vi "2017RefLoopPulseGen_Summer.vi"() -> ()   [LabVIEW 2017]
uses:
  offset_parameters.ctl
  Utility Sub VIs/pressure_temp_mixture.ctl
  Utility Sub VIs/pulse_generator_multiheater_controls.ctl
  Utility Sub VIs/valve_pid_control.ctl
  Utility Sub VIs/pulse_generator_data.ctl
  Utility Sub VIs/pulse_generator_data_charts.ctl
  Utility Sub VIs/pulse_generator_data_controls.ctl
  Input Channel Lists/test_section_physical_channels.ctl
  Input Channel Lists/float_switch_physical_channels.ctl
  Input Channel Lists/pulse_generator_input_physical_channels.ctl
  Input Channel Lists/pg_control_physical_channels.ctl
  Input Channel Lists/valve_physical_channels.ctl
  Input Channel Lists/window_heater_physical_channels.ctl
  Utility Sub VIs/windows_heater_safety_values.ctl
  Utility Sub VIs/window_heaters_control.ctl
  Utility Sub VIs/visual_loop.ctl
  Utility Sub VIs/diode_charts.ctl
  <vilib>/Utility/error.llb/DialogType.ctl
  Input Channel Lists/label_array_cluster.ctl
  Utility Sub VIs/pulse_generator_controls_multiheater_refnums.ctl
  <vilib>/Utility/sysdir.llb/System Directory Type.ctl
  <vilib>/DAQmx/read.llb/DAQmx Read (Analog 1D Wfm NChan NSamp).vi
  <vilib>/Utility/file.llb/Write Delimited Spreadsheet (string).vi
  <vilib>/DAQmx/configure/timing.llb/DAQmx Timing (Sample Clock).vi
  <vilib>/DAQmx/miscellaneous.llb/DAQmx Fill In Error Info.vi
  Utility Sub VIs/max_flow_correlation.vi
  <vilib>/addons/control/pid/autopid.llb/PID Autotuning.vi
  Stop_Global_Variable.vi
  <resource>/objmgr/daqmx.rc
  <vilib>/dex/Stream Element Allocation Mode.ctl
panel:
  out "notifier out":refnum<notifier>
  out "Float 5":bool
  out "Float 4":bool
  out "Float 3":bool
  out "Float 2":bool
  out "Float 1":bool
  out "Pulse Generator":u8(slide) scale=0.0..100.0 scale format="%.0f%"
  out "Valve Voltage Output":dbl[](array[numeric])
  out "dataQueue":refnum<queue>
  out "autoOffsetPsatQueue":refnum<queue>
  out "start time":timestamp
  out "Seconds Since\nSession Start":dbl
  out "Time Stamp":timestamp format="%<%H:%M:%S%1u>T"
  out "Data Labels":string[][](array[string])
  in  "Tab Control":T1(tab)
  in  "Tabulated/Visualized":enum32{"Tabulated", "Visualized"}(tab)
  in  "Zero Pressure Offsets":bool
  in  "Zero Temp Offsets":bool
  out "Pressure/Temperature/Mixture Properties":T2
  in  "Auto Offset":bool
  in  "Offset Parameters":T3
  out "Auto Offset Progress":u32(slide) scale=0.0..20.0
  out "# of Datasets Processed":i32
  out "Visual Loop Display":T4
  in  "Vapor PID Control":T5={"proportional gain (Kc)"=7.1567, "integral time (Ti, min)"=4.7515, "derivative time (Td, min)"=0.0, "Valve Voltage [V]"=1.0, "Min % Open"=2.0, "Max % Open"=10.0, "Reinitialize?"=FALSE, "Valve On/Off"=FALSE, "Mode"=FALSE, "Full Flow Rate"=-0.0, "Flow Set Point [g/s]"=0.0, "AutoTune"=FALSE, "Flow"={"Flow rate [g/s]"=0.0, "Line Density [g/cm^3]"=0.0}} {"Flow Set Point [g/s]" format="%.2f"; "Full Flow Rate" format="%.2f"; "Max % Open" min=0.0 max=100.0 format="%.2f"; "Min % Open" min=0.0 max=100.0 format="%.2f"; "Valve Voltage [V]" min=1.0 max=5.0 step=0.01 format="%.4f"; "derivative time (Td, min)" format="%.3f"; "integral time (Ti, min)" format="%.3f"; "proportional gain (Kc)" format="%.3f"}
  in  "Liquid PID Control":T5={"proportional gain (Kc)"=7.157, "integral time (Ti, min)"=4.752, "derivative time (Td, min)"=0.0, "Valve Voltage [V]"=1.0, "Min % Open"=2.0, "Max % Open"=3.0, "Reinitialize?"=FALSE, "Valve On/Off"=FALSE, "Mode"=FALSE, "Full Flow Rate"=0.0, "Flow Set Point [g/s]"=0.0, "AutoTune"=FALSE, "Flow"={"Flow rate [g/s]"=0.0, "Line Density [g/cm^3]"=0.0}} {"Flow Set Point [g/s]" format="%.2f"; "Full Flow Rate" format="%.2f"; "Max % Open" min=0.0 max=100.0 format="%.2f"; "Min % Open" min=0.0 max=100.0 format="%.2f"; "Valve Voltage [V]" min=1.0 max=5.0 step=0.01 format="%.4f"; "derivative time (Td, min)" format="%.3f"; "integral time (Ti, min)" format="%.3f"; "proportional gain (Kc)" format="%.3f"}
  out "Vapor Mass Flow Rate":T6(graph)
  out "Liquid Mass Flow Rate":T6(graph)
  in  "Pulse Generator Offsets":T7
  out "Measurements Data":T8={"PG Abs Pressure"=119484.80284900061, "Vapor Temperature"=19.805676371442082, "Liquid Temperature"=19.52526901660894, "TS Temperature W1"=121.24568157832624, "TS Temperature W7"=119.96937909943745, "TS Abs Pressure W1"=121.24568157832624, "TS Abs Pressure W7"=119.96937909943745, "W1-4 dP[Pa]"=19.52526901660894, "W1-7 dP[Pa]"=119.96937909943745, "W1-7 dP[Pa] Fast"=119.96937909943745, "PG Pitot dP [Pa]"=119.96937909943745, "Vapor Line Pitot dP [Pa]"=119.96937909943745, "Vapor Sat Pressure"=121.24568157832624, "Liquid Sat Pressure"=119.96937909943745, "PG Mass Flow Rate"=nan, "Vapor Line Mass Flow"=119.96937909943745}
  out "Pulse Generator Charts":T9={"Vapor Mass Flow Rates"={"max value"=119484.80284900061, "max value"=11360.460004869077}, "Test Section Thermocouples"={"max value"=0.0, "max value"=0.0, "max value"=0.0}, "Pulse Generator Abs Pressure"=[], "Test Section Saturation Pressures"={"max value"=0.0, "max value"=0.0}}
  out "Diode Charts":T10={"Diodes"={0.3021955968100006, 0.3584869363750005}, "Intensity Ratio"=0.8429751997821322, "TS Window 1 Temperatures"={"Average"=20.97750879446322, "T Sat [C]"=14.276809363087821}}
  in  "Commit Settings":bool
  in  "Settings Subpanel":T11(tab)
  in  "Input":T15={"Control Input Physical Channels"={"Vapor Mass Flow Current"="cDAQ1Mod2/ai5", "Vapor Line Density Current"="cDAQ1Mod2/ai6", "Liquid Mass Flow Current"="cDAQ1Mod2/ai3", "Liquid Line Density Current"="cDAQ1Mod2/ai4", "Vapor Tank Pressure"="cDAQ1Mod5/ai1", "Liquid Tank Pressure"="cDAQ1Mod5/ai2", "Separator Pressure"="cDAQ1Mod5/ai0", "Liquid Inlet Pressure"="cDAQ1Mod5/ai4", "Vapor Inlet Pressure"="cDAQ1Mod5/ai3", "Vapor Tank Temperature"="cDAQ1Mod6/ai1", "Vapor Inlet Temperature"="cDAQ1Mod7/ai2", "Liquid Tank Temperature"="cDAQ1Mod6/ai2", "Liquid Inlet Temperature"="cDAQ1Mod7/ai3", "Separator Temperature"="cDAQ1Mod6/ai0", "Lower Dev Section Pressure"="cDAQ1Mod5/ai6", "Test Section Temperature"="cDAQ1Mod6/ai10", "Upper Dev Section Temperature"="cDAQ1Mod6/ai3", "Upper Dev Section Pressure"="cDAQ1Mod5/ai5", "Atmospheric Pressure"="cDAQ1Mod5/ai8", "Mixing Tee dP"="cDAQ1Mod5/ai9", "PG inlet-Mixing Tee Pressure"="cDAQ1Mod5/ai10", "Test Section Pressure"="cDAQ1Mod5/ai7", "PG inlet-Mixing Tee Temperature"="cDAQ1Mod7/ai6"}, "Float Switch Physical Channels"={"Float Line 1"="Input/port0/line0", "Float Line 2"="Input/port0/line1", "Float Line 3"="Input/port0/line2", "Float Line 4"="Input/port0/line3", "Float Line 5"="Input/port0/line4"}, "Measurement Input Physical Channels"={"PG Absolute Pressure"="cDAQ1Mod5/ai11", "Pitot dP"="cDAQ1Mod2/ai7", "PG Temperature 1"="cDAQ1Mod7/ai4", "PG Temperature 2"="cDAQ1Mod7/ai5", "dP Windows 1 to 7"="cDAQ1Mod2/ai2", "dP Windows 1 to 4"="cDAQ1Mod2/ai1", "Camera Voltage"="cDAQ1Mod8/ai0", "dP Windows 1 to 4 F"="cDAQ1Mod2/ai0", "TS Temperature W1"="cDAQ1Mod6/ai4", "TS Temperature W7"="cDAQ1Mod6/ai5", "TS Abs Pressure W1"="cDAQ1Mod5/ai12", "TS Abs Pressure W7"="cDAQ1Mod5/ai13", "Main Diode"="cDAQ1Mod8/ai1", "Temperature Diode"="cDAQ1Mod8/ai2", "TS Exterior Temp"="cDAQ1Mod6/ai6", "DS Exterior Temp"="cDAQ1Mod6/ai7", "Vapor Line Pitot dP"=""}, "Float Switch Line Mode"=TRUE}
  in  "Output":T19={"Pulse Generator Control Physical Channels"={"1000W 1"="Output/port0/line1", "1000W 2"="Output/port0/line2", "1000W 3"="Output/port0/line3", "500W 1"="Output/port0/line4", "250W 1"="Output/port0/line5", "150W 1"="Output/port0/line6", "Counter Line"="cDAQ1Mod1/ctr0", "Direction Line"="cDAQ1Mod1/port0/line1"}, "Proportional Valve Physical Channels"={"Vapor Valve"="cDAQ1Mod3/ao1", "Liquid Valve"="cDAQ1Mod3/ao2", "PG Valve"="cDAQ1Mod3/ao0"}, "Window Heaters Physical Channels"={"On/Off"="cDAQ1Mod4/ao0"}, "Diode Communication"={"URL"="", "Serial"=""}}
  in  "Safety":T21={"Pulse Generator Heater Safety Values"={"Absolute Pulse Generator Pressure Limit"=250000.0, "Seconds Allowed Pulse Generator Excess Pressure"=60.0, "Absolute Pulse Generator Temperature Limit"=35.0}, "Window Heater Safety Values"={"Minimum Test Section Mass Flow "=1.0}}
  in  "Generate MATLAB Parsing Script":bool
  in  "Open Brians VI":bool
  in  "Run Log":T22(array[cluster])
  out "System Running":bool
  out "error out":errorcluster
  out "Loop Time [ms]":u32
  in  "Stop":bool
  in  "Tab Control 2":enum32{"Controls", "Offsets"}(tab)
  in  "Pulse Train, Steam Heater Controls":T23={"Start Pulse"=FALSE, "Stop Pulse"=FALSE, "Pulse Gen\nActive?"=FALSE, "Frequency (Hz)"=3000.0, "Duty Cycle"=0.5, "Idle State"=10214, "Steps"=1000, "Stepper Motor Direction"=FALSE, "Heaters"=FALSE, "Heater ON?"=FALSE, "1000-1"=FALSE, "1000-2"=FALSE, "1000-3"=FALSE, "500-1"=FALSE, "250-1"=FALSE, "150-1"=FALSE, "Valve Voltage [V]"=1.0, "Valve On/Off"=FALSE, "Power [W]"=1.0} {"Power [W]" min=1.0 max=5.0 format="%.2f"; "Valve Voltage [V]" min=1.0 max=5.0 format="%.2f"; "Frequency (Hz)" min=1.0 step=500.0; "Duty Cycle" min=0.1 max=0.99 step=0.1; "Idle State" items=["High"=10192, "Low"=10214]}
  in  "Window Heaters Control":T24
  in  "Data Saving Parameters":T25={"Sampling\nFrequency"=1000.0, "Recording Duration [s]"=10.0, "Data Index"=0, "Data Prefix"="", "Data Folder"=path "C:/Users/rmorse/Desktop/testdata", "Record Data"=FALSE, "Data Recording Progress"=0, "Notes: "=""} {"Data Recording Progress" scale=0.0..10000.0}
  in  "Offsets":T26(array[cluster])
  # "Saturation\nPressure [Pa]"
  # "Saturation\nTemperature [C]"
  # "Pressure [Pa]"
  # "Temperature [C]"
  # "Liquid Tank"
  # "Separator"
  # "Liquid Inlet"
  # "Vapor Tank"
  # "Vapor Inlet"
  # "Test Section"
  # "Upper Dev Section"
  # "Lower Dev Section"
  # "Pulse Gen"
  # "Test Section"
  # "Normal: NC\nInvert: NO\nSwitch 0 is inverted"
  # "NI-9401 Counter & DIO (pin) Chart"
  # "Default Pins used by Counter:\n     SRC: P-Gen Counter Timebase, A-input  \n     GATE: P-Gen Trigger, Z-input\n     AUX: B-input \n     OUT: P_Gen Output\nMore info:  Programs»National Instruments»NI-DAQ»NI-DAQmx Key Concepts»Counters"
  # "0"
  # "1"
  # "2"
  # "3"
  # "7 (25)"
  # "6 (23)"
  # "4 (20)"
  # "5 (22)"
  # "3 (19)"
  # "2 (17)"
  # "0 (14)"
  # "1 (16)"
  # "4 (20)"
  # "5 (22)"
  # "6 (23)"
  # "7 (25)"
  # "0 (14)"
  # "1 (16)"
  # "2 (17)"
  # "3 (19)"
  # "COUNTER"
  # "SRC"
  # "GATE"
  # "AUX"
  # "OUT"
  # "Heater Switches"
  # "PG Valve"
  # "Current Nominal Power"
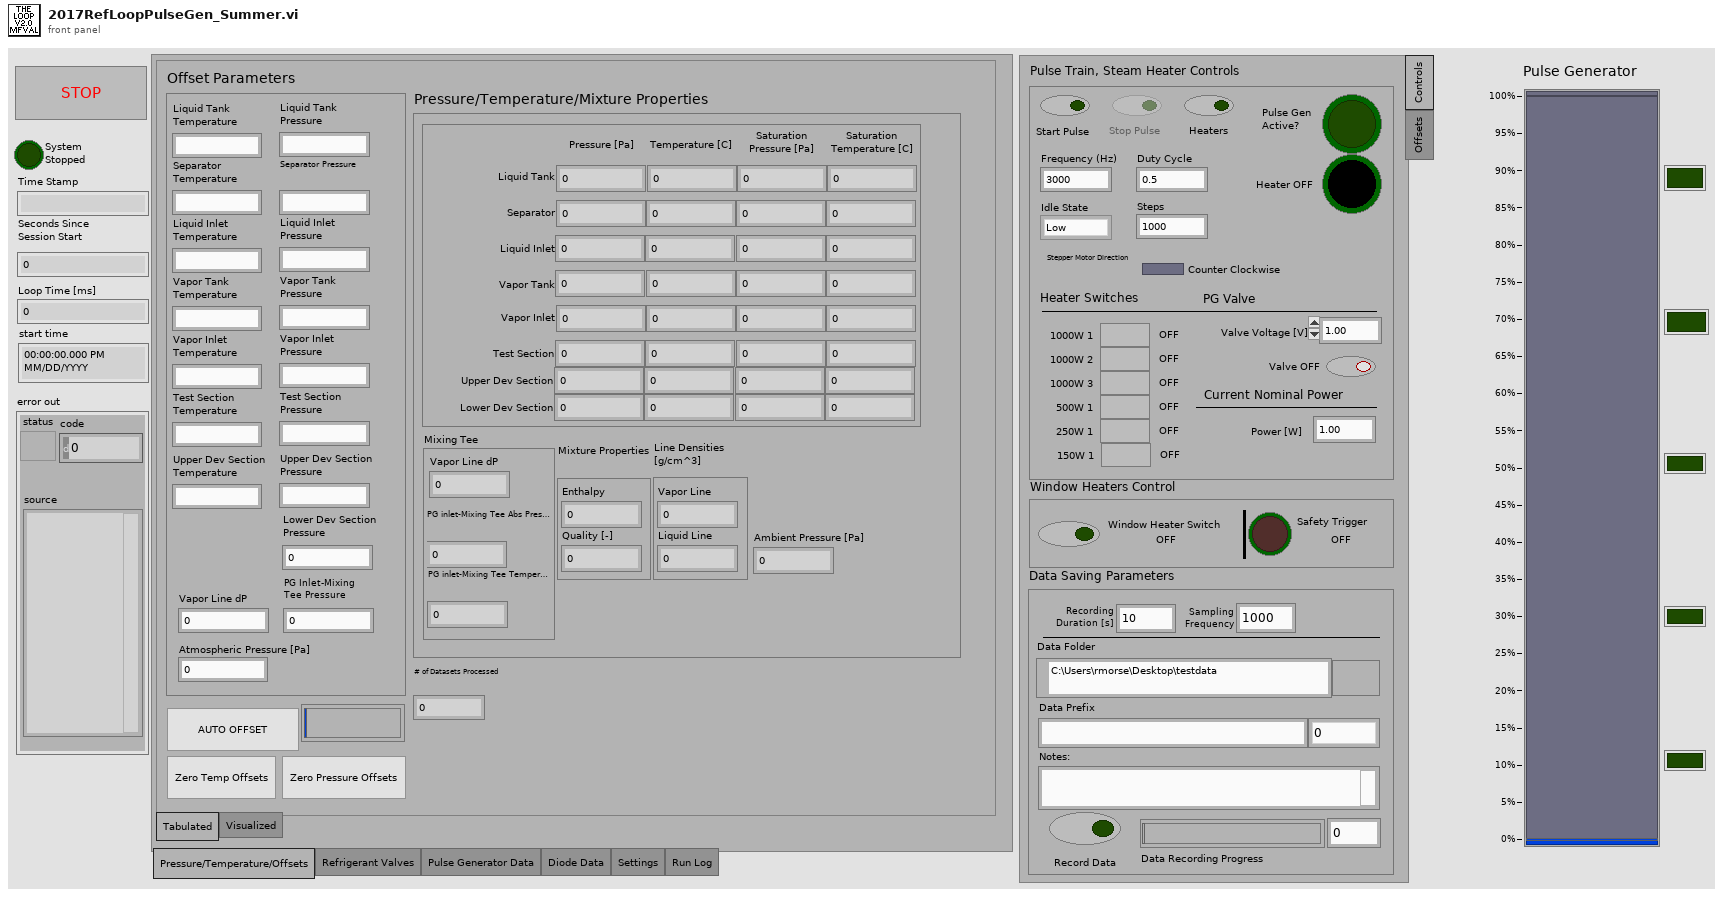
[diagram p1: front panel]
types:
  T1 = enum32{"Pressure/Temperature/Offsets", "Refrigerant Valves", "Pulse Generator Data", "Diode Data", "Settings", "Run Log"}
  T2 = typedef "pressure_temp_mixture.ctl" = cluster{"Line Densities\n[g/cm^3]":cluster{"Vapor Line":dbl, "Liquid Line":dbl}, "Mixture Properties":cluster{"Enthalpy":dbl, "Quality [-]":dbl}, "Component PTs":cluster{"Liquid Tank P":dbl, "Liquid Tank T":dbl, "Liquid Tank Sat P":dbl, "Liquid Tank Sat T":dbl, "Separator P":dbl, "Separator T":dbl, "Separator Sat P":dbl, "Separator Sat T":dbl, "Liquid Inlet P":dbl, "Liquid Inlet T":dbl, "Liquid Inlet Sat P":dbl, "Liquid Inlet Sat T":dbl, "Vapor Tank P":dbl, "Vapor Tank T":dbl, "Vapor Tank Sat P":dbl, "Vapor Tank Sat T":dbl, "Vapor Inlet P":dbl, "Vapor Inlet T":dbl, "Vapor Inlet Sat P":dbl, "Vapor Inlet Sat T":dbl, "Test Section P":dbl, "Test Section T":dbl, "Test Section Sat P":dbl, "Test Section Sat T":dbl, "Upper Dev Section P":dbl, "Upper Dev Section T":dbl, "Upper Dev Section Sat P":dbl, "Upper Dev Section Sat T":dbl, "Lower Dev Section P":dbl, "Lower Dev Section T":dbl, "Lower Dev Section Sat P":dbl, "Lower Dev Section Sat T":dbl}, "Ambient Pressure [Pa]":dbl, "Mixing Tee":cluster{"Vapor Line dP":dbl, "PG inlet-Mixing Tee Abs Pressure":dbl, "PG inlet-Mixing Tee Temperature":dbl}}
  T3 = typedef "offset_parameters.ctl" = cluster{"Liquid Tank\nPressure":dbl, "Liquid Tank\nTemperature":dbl, "Separator Pressure":dbl, "Separator \nTemperature":dbl, "Liquid Inlet\nPressure":dbl, "Liquid Inlet\nTemperature ":dbl, "Vapor Tank\nPressure ":dbl, "Vapor Tank\nTemperature ":dbl, "Vapor Inlet\nPressure":dbl, "Vapor Inlet \nTemperature":dbl, "Test Section\nPressure":dbl, "Test Section\nTemperature":dbl, "Upper Dev Section\nPressure":dbl, "Upper Dev Section\nTemperature":dbl, "Lower Dev Section\nPressure":dbl, "PG Inlet-Mixing Tee Pressure":dbl, "Vapor Line dP":dbl, "Atmospheric Pressure [Pa]":dbl}
  T4 = typedef "visual_loop.ctl" = cluster{"VpTkTemp":dbl, "VpTkPres":dbl, "LiqTkTemp":dbl, "LiqTkPres":dbl, "PGVapTemp":dbl, "PgPres":dbl, "VapInTemp":dbl, "VapInPres":dbl, "SepTemp":dbl, "SepPres":dbl, "TSInTemp":dbl, "TSInPres":dbl, "LiqInTemp":dbl, "LiqInPres":dbl, "DevTemp":dbl, "DevPres":dbl, "TSTemp":dbl, "TSPres":dbl, "Win1-4dP":dbl, "Win1-7dP":dbl, "LiqMass":dbl, "VpMass":dbl, "PGMass":dbl, "PGLiqTemp":dbl}
  T5 = typedef "valve_pid_control.ctl" = cluster{"proportional gain (Kc)":dbl, "integral time (Ti, min)":dbl, "derivative time (Td, min)":dbl, "Valve Voltage [V]":dbl, "Min % Open":dbl, "Max % Open":dbl, "Reinitialize?":bool, "Valve On/Off":bool, "Mode":bool, "Full Flow Rate":dbl, "Flow Set Point [g/s]":dbl, "AutoTune":bool, "Flow":cluster{"Flow rate [g/s]":dbl, "Line Density [g/cm^3]":dbl}}
  T6 = cluster{"Flow Set Point [g/s]":dbl, "Flow rate [g/s]":dbl}
  T7 = typedef "pulse_generator_data_controls.ctl" = cluster{"PG Pitot dP Offset":dbl, "PG Abs Offset":dbl, "W1-7 dP Offset":dbl, "W1-4 dP Offset ":dbl, "TS Abs 1 Offset":dbl, "W1-4 Fast dP Offset":dbl, "TS Abs 2 Offset":dbl, "Vapor Line Pitot dP Offset":dbl}
  T8 = typedef "pulse_generator_data.ctl" = cluster{"PG Abs Pressure":dbl, "Vapor Temperature":dbl, "Liquid Temperature":dbl, "TS Temperature W1":dbl, "TS Temperature W7":dbl, "TS Abs Pressure W1":dbl, "TS Abs Pressure W7":dbl, "W1-4 dP[Pa]":dbl, "W1-7 dP[Pa]":dbl, "W1-7 dP[Pa] Fast":dbl, "PG Pitot dP [Pa]":dbl, "Vapor Line Pitot dP [Pa]":dbl, "Vapor Sat Pressure":dbl, "Liquid Sat Pressure":dbl, "PG Mass Flow Rate":dbl, "Vapor Line Mass Flow":dbl}
  T9 = typedef "pulse_generator_data_charts.ctl" = cluster{"Vapor Mass Flow Rates":cluster{"max value":dbl, "max value":dbl}, "Test Section Thermocouples":cluster{"max value":dbl, "max value":dbl, "max value":dbl}, "Pulse Generator Abs Pressure":dbl[], "Test Section Saturation Pressures":cluster{"max value":dbl, "max value":dbl}}
  T10 = typedef "diode_charts.ctl" = cluster{"Diodes":cluster{dbl, dbl}, "Intensity Ratio":dbl, "TS Window 1 Temperatures":cluster{"Average":dbl, "T Sat [C]":dbl}}
  T11 = enum32{"Input", "Output", "Safety", "Other Functions"}
  T12 = typedef "test_section_physical_channels.ctl" = cluster{"Vapor Mass Flow Current":tag, "Vapor Line Density Current":tag, "Liquid Mass Flow Current":tag, "Liquid Line Density Current":tag, "Vapor Tank Pressure":tag, "Liquid Tank Pressure":tag, "Separator Pressure":tag, "Liquid Inlet Pressure":tag, "Vapor Inlet Pressure":tag, "Vapor Tank Temperature":tag, "Vapor Inlet Temperature":tag, "Liquid Tank Temperature":tag, "Liquid Inlet Temperature":tag, "Separator Temperature":tag, "Lower Dev Section Pressure":tag, "Test Section Temperature":tag, "Upper Dev Section Temperature":tag, "Upper Dev Section Pressure":tag, "Atmospheric Pressure":tag, "Mixing Tee dP":tag, "PG inlet-Mixing Tee Pressure":tag, "Test Section Pressure":tag, "PG inlet-Mixing Tee Temperature":tag}
  T13 = typedef "float_switch_physical_channels.ctl" = cluster{"Float Line 1":tag, "Float Line 2":tag, "Float Line 3":tag, "Float Line 4":tag, "Float Line 5":tag}
  T14 = typedef "pulse_generator_input_physical_channels.ctl" = cluster{"PG Absolute Pressure":tag, "Pitot dP":tag, "PG Temperature 1":tag, "PG Temperature 2":tag, "dP Windows 1 to 7":tag, "dP Windows 1 to 4":tag, "Camera Voltage":tag, "dP Windows 1 to 4 F":tag, "TS Temperature W1":tag, "TS Temperature W7":tag, "TS Abs Pressure W1":tag, "TS Abs Pressure W7":tag, "Main Diode":tag, "Temperature Diode":tag, "TS Exterior Temp":tag, "DS Exterior Temp":tag, "Vapor Line Pitot dP":tag}
  T15 = cluster{"Control Input Physical Channels":T12, "Float Switch Physical Channels":T13, "Measurement Input Physical Channels":T14, "Float Switch Line Mode":bool}
  T16 = typedef "pg_control_physical_channels.ctl" = cluster{"1000W 1":tag, "1000W 2":tag, "1000W 3":tag, "500W 1":tag, "250W 1":tag, "150W 1":tag, "Counter Line":tag, "Direction Line":tag}
  T17 = typedef "valve_physical_channels.ctl" = cluster{"Vapor Valve":tag, "Liquid Valve":tag, "PG Valve":tag}
  T18 = typedef "window_heater_physical_channels.ctl" = cluster{"On/Off":tag}
  T19 = cluster{"Pulse Generator Control Physical Channels":T16, "Proportional Valve Physical Channels":T17, "Window Heaters Physical Channels":T18, "Diode Communication":cluster{"URL":string, "Serial":refnum<visa-resource-name>}}
  T20 = typedef "windows_heater_safety_values.ctl" = cluster{"Minimum Test Section Mass Flow ":dbl}
  T21 = cluster{"Pulse Generator Heater Safety Values":cluster{"Absolute Pulse Generator Pressure Limit":dbl, "Seconds Allowed Pulse Generator Excess Pressure":dbl, "Absolute Pulse Generator Temperature Limit":dbl}, "Window Heater Safety Values":T20}
  T22 = cluster{"File Number":string, "Entry Content":string}[]
  T23 = typedef "pulse_generator_multiheater_controls.ctl" = cluster{"Start Pulse":bool, "Stop Pulse":bool, "Pulse Gen\nActive?":bool, "Frequency (Hz)":dbl, "Duty Cycle":dbl, "Idle State":i32, "Steps":i32, "Stepper Motor Direction":bool, "Heaters":bool, "Heater ON?":bool, "1000-1":bool, "1000-2":bool, "1000-3":bool, "500-1":bool, "250-1":bool, "150-1":bool, "Valve Voltage [V]":dbl, "Valve On/Off":bool, "Power [W]":dbl}
  T24 = typedef "window_heaters_control.ctl" = cluster{"Window Heater Switch":bool, "Safety Trigger":bool}
  T25 = cluster{"Sampling\nFrequency":dbl, "Recording Duration [s]":dbl, "Data Index":i32, "Data Prefix":string, "Data Folder":path, "Record Data":bool, "Data Recording Progress":u32, "Notes: ":string}
  T26 = cluster{"Channel":string, "Offset":dbl, "Output Unit":enum16{"psi", "Pa", "inH2O", "inHg", "C", "K", "g/s", "g/cm3", "Volt", "Amp", ""}}[]
  T27 = enum32{"Pressure/Temperature/Offsets", "Refrigerant Valves", "Pulse Generator Data", "Diode Data", "Settings"}
  T28 = enum8{"Enabled", "Disabled", "Disabled and Grayed Out"}
  T29 = cluster{"max value":dbl, "max value":dbl, "max value":dbl}[]
  T30 = enum32{"Pressure/Temperature/Offsets", "Refrigerant Valves", "Pulse Generator Data", "Settings"}
  T31 = cluster{"Channel Name":string, "Label":string, "Offset":dbl, "Raw":dbl[], "Processed":dbl[], "Converted":dbl[], "Average":dbl}
  T32 = typedef "label_array_cluster.ctl" = cluster{"Label Array":string[]}
  T33 = enum32{"Invalid", "Standard", "Closed", "Hidden", "Minimized", "Maximized"}
  T34 = cluster{"Entry Content":string, "File Number":string}
  T35 = typedef "DialogType.ctl" = u16
  T36 = cluster{"Flow Set Point [g/s]":dbl, "Flow rate [g/s]":dbl}[]
  T37 = typedef "analog_data_channel_pkg.ctl" = cluster{"Analog Input Channel":T38, "Analog Data":T39}
  T38 = typedef "input_channel.ctl" = cluster{"Channel Name":string, "Physical Channel":tag, "Sensor Type":enum16{"Absolute Pressure", "Gauge Pressure", "Differential Pressure", "Temperature", "Mass Flow Rate", "Density", "Other"}, "Signal Type":enum16{"Voltage", "Current", "Temperature"}, "Terminal Configuration":i32, "Minimum Value":dbl, "Maximum Value":dbl, "TC Type":i32, "Sensor Min":dbl, "Sensor Max":dbl, "Sensor Offset":dbl, "Sensor Unit":enum16{"psi", "Pa", "inH2O", "inHg", "C", "K", "g/s", "g/cm3", "Volt", "Amp", ""}, "Output Unit":enum16{"psi", "Pa", "inH2O", "inHg", "C", "K", "g/s", "g/cm3", "Volt", "Amp", ""}, "Unit Conversion":dbl, "Active":bool, "Input Type":enum16{"DAQ", "Add-On"}}
  T39 = typedef "analog_data.ctl" = cluster{"Label":string, "Offset":dbl, "Raw":dbl[], "Converted":dbl[], "Average":dbl, "Formula To Output":string, "Formula From Output":string}
  T40 = enum16{"psi", "Pa", "inH2O", "inHg", "C", "K", "g/s", "g/cm3", "Volt", "Amp", ""}
  T41 = cluster{"Label":string, "Offset":dbl, "Output Unit":enum16{"psi", "Pa", "inH2O", "inHg", "C", "K", "g/s", "g/cm3", "Volt", "Amp", ""}}
  T42 = typedef "index_array_cluster.ctl" = cluster{"Index Array":i32[]}
  T43 = typedef "Stream Element Allocation Mode.ctl" = u32
  T44 = typedef "pulse_generator_controls_multiheater_refnums.ctl" = cluster{"Start Pulse":refnum<vi>, "Stop Pulse":refnum<vi>, "Heaters":refnum<vi>, "Counter":refnum<vi>, "Frequency (Hz)":refnum<vi>, "Duty Cycle":refnum<vi>, "Idle State":refnum<vi>, "Pulse Generator Active":refnum<vi>, "Stepper Motor Direction":refnum<vi>, "Steps":refnum<vi>, "Direction Line":refnum<vi>, "1000-1 Line":refnum<vi>, "1000-2 Line":refnum<vi>, "1000-3 Line":refnum<vi>, "500-1 Line":refnum<vi>, "250-1 Line":refnum<vi>, "1000-1":refnum<vi>, "1000-2":refnum<vi>, "1000-3":refnum<vi>, "500-1":refnum<vi>, "250-1":refnum<vi>, "150-1":refnum<vi>, "Heater ON?":refnum<vi>, "150-1 Line":refnum<vi>, "Power":refnum<vi>}
  T45 = cluster{"Liquid Tank P":dbl, "Liquid Tank T":dbl, "Liquid Tank Sat P":dbl, "Liquid Tank Sat T":dbl, "Separator P":dbl, "Separator T":dbl, "Separator Sat P":dbl, "Separator Sat T":dbl, "Liquid Inlet P":dbl, "Liquid Inlet T":dbl, "Liquid Inlet Sat P":dbl, "Liquid Inlet Sat T":dbl, "Vapor Tank P":dbl, "Vapor Tank T":dbl, "Vapor Tank Sat P":dbl, "Vapor Tank Sat T":dbl, "Vapor Inlet P":dbl, "Vapor Inlet T":dbl, "Vapor Inlet Sat P":dbl, "Vapor Inlet Sat T":dbl, "Test Section P":dbl, "Test Section T":dbl, "Test Section Sat P":dbl, "Test Section Sat T":dbl, "Upper Dev Section P":dbl, "Upper Dev Section T":dbl, "Upper Dev Section Sat P":dbl, "Upper Dev Section Sat T":dbl, "Lower Dev Section P":dbl, "Lower Dev Section T":dbl, "Lower Dev Section Sat P":dbl, "Lower Dev Section Sat T":dbl}
  T46 = cluster{"Channel":string, "Offset":dbl, "Output Unit":enum16{"psi", "Pa", "inH2O", "inHg", "C", "K", "g/s", "g/cm3", "Volt", "Amp", ""}}
  T47 = typedef "System Directory Type.ctl" = i32
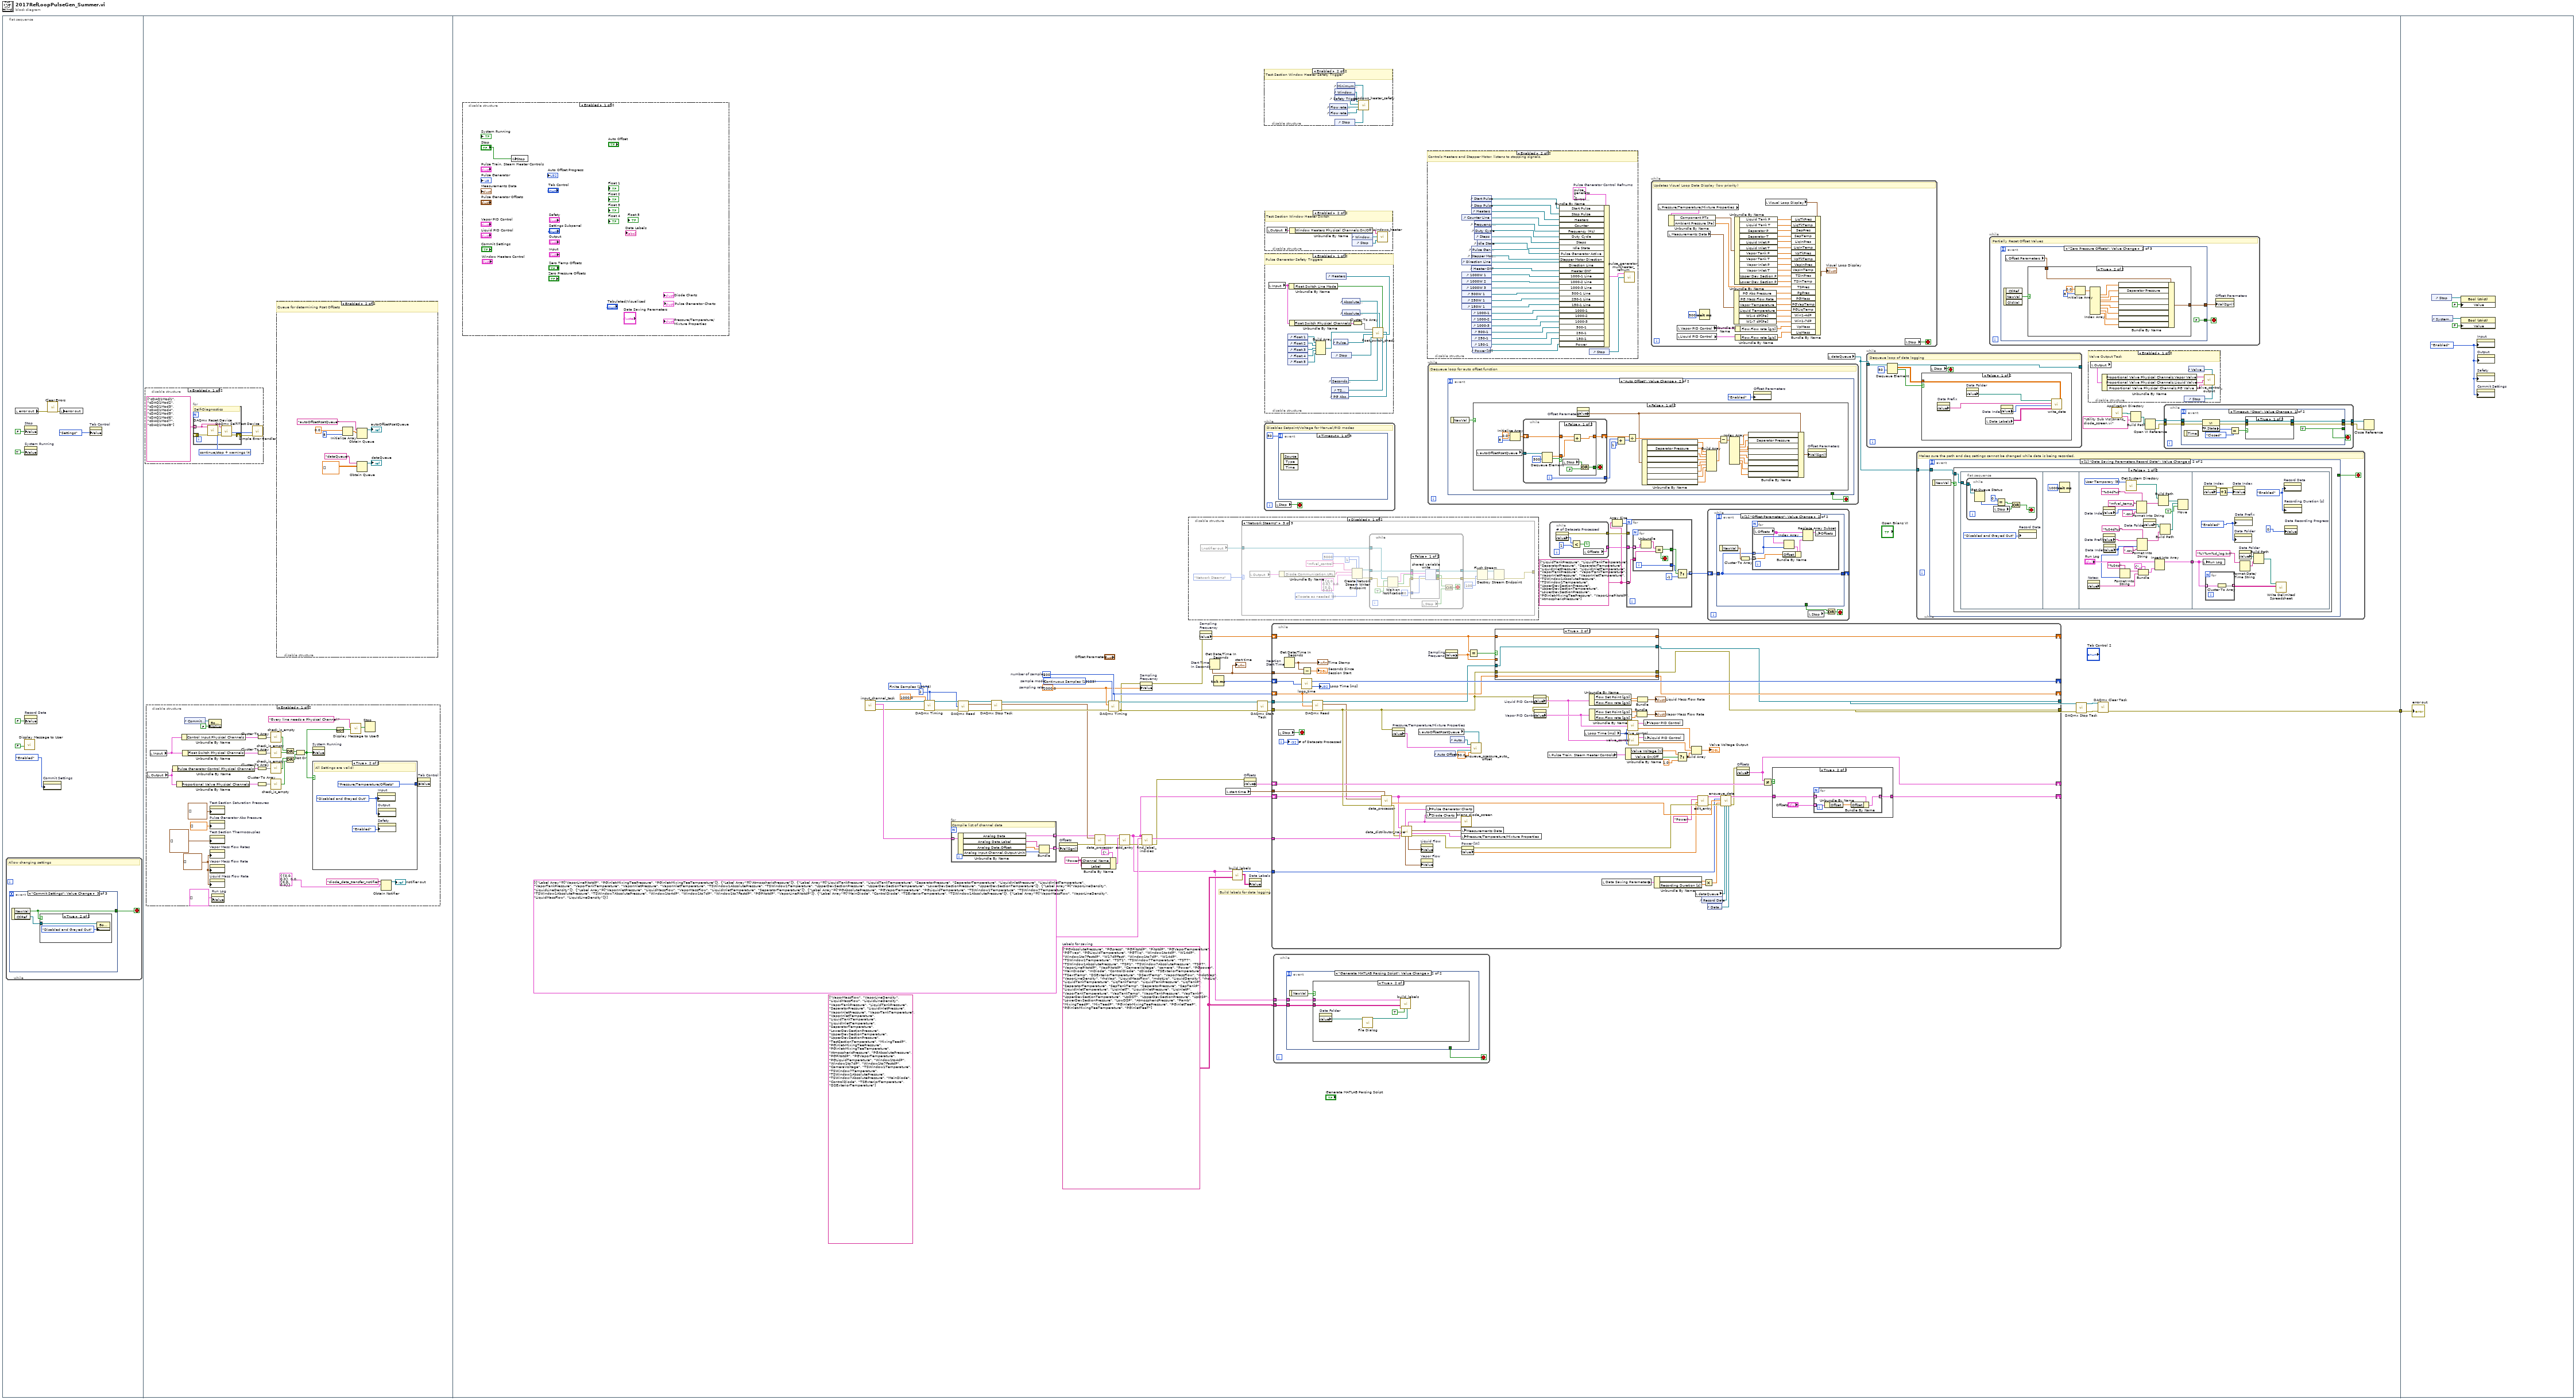
[diagram p0: block diagram]
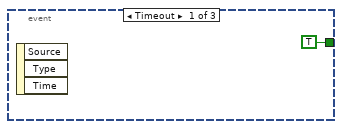
[diagram p2: hidden frame]
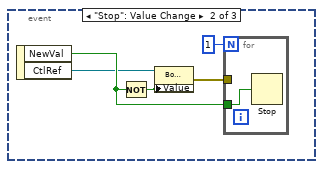
[diagram p3: hidden frame]
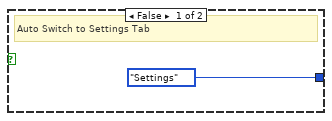
[diagram p6: hidden frame]
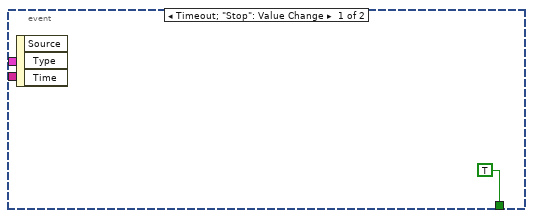
[diagram p9: hidden frame]
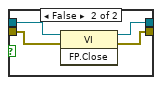
[diagram p11: hidden frame]
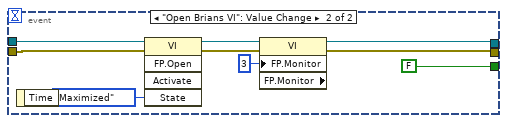
[diagram p12: hidden frame]
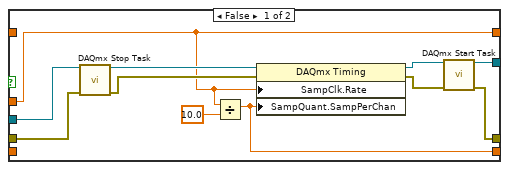
[diagram p14: hidden frame]
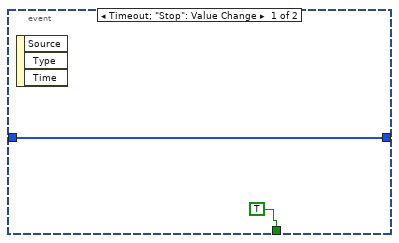
[diagram p15: hidden frame]
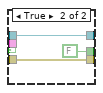
[diagram p18: hidden frame]
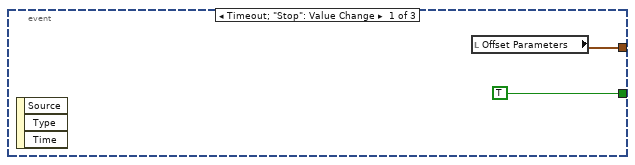
[diagram p20: hidden frame]
diagram:
  n1 = flat-sequence {
    tunnel: [w130] -> w1
    tunnel: w1 -> [w628]
    frame #0 {
      n2 = while {
        stop <- w10 stop-if-true
        # "Allow changing settings"
        n3 = event shown="[2] \"Commit Settings\": Value Change" {
          selector: _ -> [_ _ _]
          dyn-events: _ -> [_ _ _]
          timeout: _ -> [_ _ _]
          tunnel: [TRUE ("NewVal") _ w18] -> w10
          event Timeout {
            n4 = event-data() -> ()  [unwired: 1 in, 3 out]
          }
          event "Stop": Value Change {
            n5 = event-data() -> ("NewVal"=w16:bool, "CtlRef"=w15:refnum<vi>)  [unwired: 1 in]
            n6 = Not(x=w16) -> (.not. x?=w14:bool)
            n7 = property class="Bool (strict)"(reference=w15, "Value"=w14) -> (error out=w13:errorcluster)  [unwired: 1 in, 1 out]
            n8 = for {
              N: 1 -> [_]
              tunnel: w16 -> [w17]
              tunnel: w13 -> [_]
              n9 = Stop(stop? (T)=w17) -> ()
            }
          }
          event "Commit Settings": Value Change {
            n10 = event-data() -> ("NewVal"=w18:bool, "CtlRef"=w19:refnum<vi>)  [unwired: 1 in]
            n11 = case shown="True" w18 {
              tunnel: w19 -> [_ w21]
              frame False {
              }
              frame True {
                n12 = property class="Bool (strict)"(reference=w21, "DisabledEnum"=T28."Disabled and Grayed Out" ("Disabled")) -> ()  [unwired: 1 in, 2 out]
              }
            }
          }
        }
      }
      n13 = local read "error out"() -> (w9:errorcluster)
      n14 = call "Display Message to User"("Enable"=FALSE) -> ()  [unwired: 9 in, 2 out]
      n15 = property on="Stop" class="Bool (strict)"("Value"=FALSE) -> ()  [unwired: 2 in, 2 out]
      n16 = property on="System Running" class="Bool (strict)"("Value"=TRUE) -> ()  [unwired: 2 in, 2 out]
      n17 = property on="Record Data" class="Bool (strict)"("Value"=FALSE) -> ()  [unwired: 2 in, 2 out]
      n18 = property on="Commit Settings" class="Bool (strict)"("DisabledEnum"=T28."Enabled" ("Disabled")) -> ()  [unwired: 2 in, 2 out]
      n19 = call <vilib>:"Clear Errors.vi"("error in (no error)"=w9) -> ("error out"=w7:errorcluster)  [unwired: 5 in, 1 out]
      n20 = local write "error out"(w7) -> ()
      n21 = property on="Tab Control" class="TabCtl (strict)"("Value"=T27."Settings" ("Tab Control")) -> ()  [unwired: 2 in, 2 out]
    }
    frame #1 {
      n22 = disable-structure shown="Enabled" {
        frame Enabled {
          w65 = T35 4 items=["no dialog", "OK message", "continue or stop message", "OK message + warnings", "continue/stop + warnings"] ("type of dialog (OK msg:1)")
          n23 = for {
            tunnel: string[] ["cDAQ1Mod1", "cDAQ1Mod2", "cDAQ1Mod3", "cDAQ1Mod4", "cDAQ1Mod5", "cDAQ1Mod6", "cDAQ1Mod7", "cDAQ1Mod8"] -> [w69] mode=indexing
            shift-right: [w71] -> w66
            shift-left: _ -> [w68]
            # "Self-Diagnostics"
            n24 = call <vilib>:"DAQmx Reset Device.vi"("device in"=w69, "error in"=w68) -> ("error out"=w70:errorcluster)  [unwired: 13 in]
            n25 = call <vilib>:"DAQmx Self-Test Device.vi"("device in"=w69, "error in"=w70) -> ("error out"=w71:errorcluster)  [unwired: 13 in]
          }
          n26 = call <vilib>:"Simple Error Handler.vi"("type of dialog (OK msg:1)"=w65, "error in (no error)"=w66) -> ()  [unwired: 3 in, 5 out]
        }
        frame Disabled {
        }
      }
      n27 = disable-structure shown="Enabled" {
        frame Enabled {
          w31 = T36 [] ("History Data")
          n28 = local read "Output"() -> (w38:T19)
          n29 = local read "Input"() -> (w44:T15)
          n30 = Unbundle By Name(w38) -> ("Pulse Generator Control Physical Channels"=w45:T16)
          n31 = Unbundle By Name(w38) -> ("Proportional Valve Physical Channels"=w43:T17)
          n32 = Unbundle By Name(w44) -> ("Control Input Physical Channels"=w47:T12)
          n33 = Unbundle By Name(w44) -> ("Float Switch Physical Channels"=w46:T13)
          n34 = control-ref of="Commit Settings"() -> (w41:refnum<vi>)
          n35 = property class="Bool (strict)"(reference=w41, "Value"=FALSE ("Commit Settings")) -> ()  [unwired: 1 in, 2 out]
          n36 = property on="Test Section Saturation Pressures" class="WFChart (strict)"("History Data"=cluster{"max value":dbl, "max value":dbl}[] []) -> ()  [unwired: 2 in, 2 out]
          n37 = property on="Pulse Generator Abs Pressure" class="WFChart (strict)"("History Data"=dbl[] []) -> ()  [unwired: 2 in, 2 out]
          n38 = property on="Test Section Thermocouples" class="WFChart (strict)"("History Data"=T29 []) -> ()  [unwired: 2 in, 2 out]
          n39 = property on="Vapor Mass Flow Rates" class="WFChart (strict)"("History Data"=w31) -> ()  [unwired: 2 in, 2 out]
          n40 = property on="Vapor Mass Flow Rate" class="WFChart (strict)"("History Data"=w31) -> ()  [unwired: 2 in, 2 out]
          n41 = property on="Liquid Mass Flow Rate" class="WFChart (strict)"("History Data"=w31) -> ()  [unwired: 2 in, 2 out]
          n42 = property on="Run Log" class="Arr (strict)"("Value"=T22 [] ("Run Log")) -> ()  [unwired: 2 in, 2 out]
          n43 = Cluster To Array(cluster=w47) -> (array=w60:tag[])
          n44 = Cluster To Array(cluster=w46) -> (array=w59:tag[])
          n45 = Cluster To Array(cluster=w45) -> (array=w56:tag[])
          n46 = Cluster To Array(cluster=w43) -> (array=w54:tag[])
          n47 = call "check_is_empty.vi"("Channels"=w60) -> ("Has Empty?"=w58:bool)
          n48 = call "check_is_empty.vi"("Channels"=w59) -> ("Has Empty?"=w57:bool)
          n49 = call "check_is_empty.vi"("Channels"=w56) -> ("Has Empty?"=w53:bool)
          n50 = call "check_is_empty.vi"("Channels"=w54) -> ("Has Empty?"=w52:bool)
          n51 = Or(x=w58, y=w57) -> (x .or. y?=w55:bool)
          n52 = Or(x=w53, y=w52) -> (x .or. y?=w51:bool)
          n53 = Not Or(1:w51, 2:w55) -> (0:w39:bool)
          n54 = property on="System Running" class="Bool (strict)"("Value"=w39) -> ()  [unwired: 2 in, 2 out]
          n55 = case shown="True" w39 {
            tunnel: [T30."Settings" ("Tab Control") T27."Pressure/Temperature/Offsets" ("Tab Control")] -> w42
            frame False {
              # "Auto Switch to Settings Tab"
            }
            frame True {
              w63 = T28."Disabled and Grayed Out" ("Disabled")
              # "All Settings are valid!"
              n56 = property on="Input" class="Clust (strict)"("DisabledEnum"=w63) -> ()  [unwired: 2 in, 2 out]
              n57 = property on="Output" class="Clust (strict)"("DisabledEnum"=w63) -> ()  [unwired: 2 in, 2 out]
              n58 = property on="Safety" class="Clust (strict)"("DisabledEnum"=T28."Enabled" ("Disabled")) -> ()  [unwired: 2 in, 2 out]
            }
          }
          n59 = Not(x=w39) -> (.not. x?=w50:bool)
          n60 = call "Display Message to User5"("Enable"=w50, "Message"="Every line needs a Physical Channel!") -> ("OK"=w48:bool)  [unwired: 8 in, 1 out]
          n61 = Stop(stop? (T)=w48) -> ()
          n62 = Obtain Notifier(name (unnamed)="diode_data_transfer_notifier", notification data type=T10 {"Diodes"={0.0, 0.0}, "Intensity Ratio"=0.0, "TS Window 1 Temperatures"={"Average"=0.0, "T Sat [C]"=0.0}} ("Diode Charts")) -> (notifier out=→"notifier out":refnum<notifier>)  [unwired: 2 in, 2 out]
          n63 = property on="Tab Control" class="TabCtl (strict)"("Value"=w42) -> ()  [unwired: 2 in, 2 out]
        }
        frame Disabled {
        }
      }
      n64 = disable-structure shown="Enabled" {
        frame Disabled {
        }
        frame Enabled {
          # "Queue for determining Psat Offsets"
          n65 = Initialize Array(0.0 ("element"), 8 ("dimension size")) -> (w29:dbl[])
          n66 = Obtain Queue(name (unnamed)="autoOffsetPsatQueue", element data type=w29) -> (queue out=→"autoOffsetPsatQueue":refnum<queue>)  [unwired: 3 in, 2 out]
          n67 = Obtain Queue(name (unnamed)="dataQueue", element data type=dbl[][] [] ("appended array")) -> (queue out=→"dataQueue":refnum<queue>)  [unwired: 3 in, 2 out]
        }
      }
    }
    frame #2 {
      w84 = "Power" ("Channel Name")
      w102 = 10178 items=["Finite Samples"=10178, "Continuous Samples"=10123, "Hardware Timed Single Point"=12522] ("sample mode")
      w98 = 2 ("samples per channel")
      w110 = string[] ["LiquidTankPressure", "LiquidTankTemperature", "SeparatorPressure", "SeparatorTemperature", "LiquidInletPressure", "LiquidInletTemperature", "VaporTankPressure", "VaporTankTemperature", "VaporInletPressure", "VaporInletTemperature", "TSWindow1AbsolutePressure", "TSWindow1Temperature", "UpperDevSectionPressure", "UpperDevSectionTemperature", "LowerDevSectionPressure", "PGinlet-MixingTeePressure", "VaporLinePitotdP", "AtmosphericPressure"] ("Array")
      w73 = string[][] [["PGAbsolutePressure", "PGpress"], ["PGPitotdP", "PitotdP"], ["PGVaporTemperature", "PGTvap"], ["PGLiquidTemperature", "PGTliq"], ["Window1to4dP", "W14dP"], ["Window1to7FastdP", "W17dPFast"], ["Window1to7dP", "W14dP"], ["TSWindow1Temperature", "TST1"], ["TSWindow7Temperature", "TST7"], ["TSWindow1AbsolutePressure", "TSP1"], ["TSWindow7AbsolutePressure", "TSP7"], ["VaporLinePitotdP", "VapPitotdP"], ["CameraVoltage", "camera"], ["Power", "PGpower"], ["MainDiode", "mDiode"], ["ControlDiode", "cDiode"], ["TSExteriorTemperature", "TSextTemp"], ["DSExteriorTemperature", "DSextTemp"], ["VaporMassFlow", "mdotVap"], ["VaporLineDensity", "rhoVap"], ["LiquidMassFlow", "mdotLiq"], ["LiquidDensity", "rhoLiq"], ["LiquidTankTemperature", "LiqTankTemp"], ["LiquidTankPressure", "LiqTankP"], ["SeparatorTemperature", "SepTankTemp"], ["SeparatorPressure", "SepTankP"], ["LiquidInletTemperature", "LiqInletT"], ["LiquidInletPressure", "LiqInletP"], ["VaporTankTemperature", "VapTankTemp"], ["VaporTankPressure", "VapTankP"], ["UpperDevSectionTemperature", "UpDST"], ["UpperDevSectionPressure", "UpDSP"], ["LowerDevSectionPressure", "LowDSP"], ["AtmosphericPressure", "Pamb"], ["MixingTeedP", "MixTeedP"], ["PGinlet-MixingTeePressure", "PGinletTeeP"], ["PGinlet-MixingTeeTemperature", "PGinletTeeT"]]  # Labels for saving
      (unwired) string[] ["VaporMassFlow", "VaporLineDensity", "LiquidMassFlow", "LiquidLineDensity", "VaporTankPressure", "LiquidTankPressure", "SeparatorPressure", "LiquidInletPressure", "VaporInletPressure", "VaporTankTemperature", "VaporInletTemperature", "LiquidTankTemperature", "LiquidInletTemperature", "SeparatorTemperature", "LowerDevSectionPressure", "UpperDevSectionTemperature", "UpperDevSectionPressure", "TestSectionTemperature", "MixingTeedP", "PGinlet-MixingTeePressure", "PGinlet-MixingTeeTemperature", "AtmosphericPressure", "PGAbsolutePressure", "PGPitotdP", "PGVaporTemperature", "PGLiquidTemperature", "Window1to4dP", "Window1to7dP", "Window1to7FastdP", "CameraVoltage", "TSWindow1Temperature", "TSWindow7Temperature", "TSWindow1AbsolutePressure", "TSWindow7AbsolutePressure", "MainDiode", "ControlDiode", "TSExteriorTemperature", "DSExteriorTemperature"] ("Array")
      w125 = 10123 items=["Finite Samples"=10178, "Continuous Samples"=10123, "Hardware Timed Single Point"=12522]  # sample mode
      w123 = 2000.0  # sampling rate
      w124 = 200  # number of samples
      # "Build labels for data logging"
      n68 = disable-structure shown="Enabled" {
        frame Enabled {
          n69 = global write "Stop_Global_Variable.vi" "Stop"("Stop") -> ()
        }
        frame Disabled {
        }
      }
      n70 = call "input_channel_task.vi"() -> ("error out"=w103:errorcluster, "Active Analog Channel-Data Packages"=w119:T37[], "task out"=w104:refnum<k21>)  [unwired: 9 in]
      n71 = call-poly <vilib>:"DAQmx Timing.vi"("task/channels in"=w104, "sample mode"=w102, "samples per channel"=w98, "rate"=1000.0, "error in"=w103) -> ("task out"=w100:refnum<k21>, "error out"=w99:errorcluster)  [unwired: 9 in]
      n72 = for {
        tunnel: w119 -> [w311] mode=indexing
        tunnel: [w310] -> w77 mode=indexing
        tunnel: [w308] -> w116 mode=indexing
        # "Compile list of channel data"
        n73 = Unbundle By Name(w311) -> ("Analog Data"=w310:T39, "Analog Data.Label"=w306:string, "Analog Data.Offset"=w309:dbl, "Analog Input Channel.Output Unit"=w307:T40)
        n74 = Bundle("Label"=w306, "Offset"=w309, "Output Unit"=w307) -> (w308:T41)  [unwired: 1 in]
      }
      n75 = call-poly <vilib>:"DAQmx Read.vi"("task/channels in"=w100, "number of samples per channel"=w98, "error in"=w99) -> ("task out"=w97:refnum<k21>, "data"=w78:waveform(dbl)[], "error out"=w96:errorcluster)  [unwired: 10 in]
      n76 = call <vilib>:"DAQmx Stop Task.vi"("task/channels in"=w97, "error in"=w96) -> ("task out"=w94:refnum<k21>, "error out"=w95:errorcluster)  [unwired: 12 in]
      n77 = property on="Offsets" class="Arr (strict)"("Val(Sgnl)"=w116) -> (error out=w80:errorcluster)  [unwired: 2 in, 1 out]
      n78 = Bundle By Name(cluster=T31 {"Channel Name"="", "Label"="", "Offset"=0.0, "Raw"=[], "Processed"=[], "Converted"=[], "Average"=0.0} ("Add-on Data"), "Channel Name"=w84, "Label"=w84) -> (w85:T31)
      n79 = call "data_processor.vi"("Active Analog Data Packages In"=w77, "data"=w78, "error in"=w80) -> ("Analog Data Array"=w83:T39[], "error out"=w82:errorcluster)  [unwired: 10 in, 1 out]
      n80 = call-poly <vilib>:"DAQmx Timing.vi"("task/channels in"=w94, "sample mode"=w125, "samples per channel"=w124, "rate"=w123, "error in"=w95) -> ("task out"=w114:refnum<k21>, "error out"=w113:errorcluster)  [unwired: 9 in]
      n81 = call "add_entry.vi"("Active Analog Data In"=w83, "Add-on Data"=w85, "error in"=w82) -> ("Active Analog Data Out"=w72:T39[], "error out"=w81:errorcluster)  [unwired: 11 in]
      n82 = property on="Sampling\nFrequency" class="DigNum (strict)"(error in=w113, "Value"=w123) -> (error out=w121:errorcluster)  [unwired: 1 in, 1 out]
      n83 = call "find_label_indicies.vi"("error in"=w81, "Array"=T32[] [{"Label Array"=["VaporLinePitotdP", "PGinlet-MixingTeePressure", "PGinlet-MixingTeeTemperature"]}, {"Label Array"=["AtmosphericPressure"]}, {"Label Array"=["LiquidTankPressure", "LiquidTankTemperature", "SeparatorPressure", "SeparatorTemperature", "LiquidInletPressure", "LiquidInletTemperature", "VaporTankPressure", "VaporTankTemperature", "VaporInletPressure", "VaporInletTemperature", "TSWindow1AbsolutePressure", "TSWindow1Temperature", "UpperDevSectionPressure", "UpperDevSectionTemperature", "LowerDevSectionPressure", "UpperDevSectionTemperature"]}, {"Label Array"=["VaporLineDensity", "LiquidLineDensity"]}, {"Label Array"=["VaporInletPressure", "LiquidMassFlow", "VaporMassFlow", "LiquidInletTemperature", "SeparatorTemperature"]}, {"Label Array"=["PGAbsolutePressure", "PGVaporTemperature", "PGLiquidTemperature", "TSWindow1Temperature", "TSWindow7Temperature", "TSWindow1AbsolutePressure", "TSWindow7AbsolutePressure", "Window1to4dP", "Window1to7dP", "Window1to7FastdP", "PGPitotdP", "VaporLinePitotdP"]}, {"Label Array"=["MainDiode", "ControlDiode", "TSExteriorTemperature", "TSWindow1AbsolutePressure"]}, {"Label Array"=["VaporMassFlow", "VaporLineDensity", "LiquidMassFlow", "LiquidLineDensity"]}], "haystack"=w72) -> ("error out"=w79:errorcluster, "Indicies"=w118:T42[])  [unwired: 6 in, 1 out]
      n84 = disable-structure shown="Disabled" {
        frame Disabled {
          n85 = local read "notifier out"() -> (w312:refnum<notifier>)
          n86 = case shown="\"Network Steams\"" enum16{"Network Steams", "Datasocket", "Serial"}."Network Steams" {
            tunnel: w312 -> [_ _ w315]
            tunnel: [_ _ w314] -> _
            frame Default {
            }
            frame "Datasocket" {
            }
            frame "Network Steams" {
              w324 = T43 0 items=["allocate as needed", "pre-allocate"] ("element allocation mode")
              n87 = local read "Output"() -> (w328:T19)
              n88 = Unbundle By Name(w328) -> ("Diode Communication.URL"=w327:string)
              n89 = Create Network Stream Writer Endpoint(5:5000 ("timeout in ms (-1)"), 6:w324, 7:1 ("writer buffer size"), 9:T10 {"Diodes"={0.0, 0.0}, "Intensity Ratio"=0.0, "TS Window 1 Temperatures"={"Average"=0.0, "T Sat [C]"=0.0}} ("Diode Charts"), 10:w327, 11:"mfval_control" ("writer name")) -> (0:w316:errorcluster, 3:w317:refnum<k21>)  [unwired: 1 in]
              n90 = while {
                tunnel: w315 -> [w336]
                tunnel: w317 -> [w339]
                tunnel: [w341] -> w319
                tunnel: w316 -> [w338]
                tunnel: [w340] -> w318
                stop <- w332 stop-if-true
                n91 = Wait on Notification(notifier=w336, ignore previous (F)=TRUE, error in (no error)=w338) -> (notification=w334:T10, timed out?=w333:bool, error out=w337:errorcluster)  [unwired: 1 in, 1 out]
                n92 = case shown="False" w333 {
                  tunnel: 80 ("timeout ms (-1)") -> [w349 _]
                  tunnel: [w348 w352] -> w341
                  tunnel: [w347 w351] -> w340
                  tunnel: w339 -> [w346 w352]
                  tunnel: [w345 FALSE] -> w331
                  tunnel: w337 -> [w344 w351]
                  tunnel: w334 -> [w343 _]
                  frame False {
                    n93 = shared-variable-write(w346, w344, w343, w349) -> (w348:refnum<k21>, w347:errorcluster, w345:bool)
                  }
                  frame True {
                  }
                }
                n94 = local read "Stop"() -> (w330:bool)
                n95 = Or(x=w331, y=w330) -> (x .or. y?=w332:bool)
              }
              n96 = Flush Stream(8:w318, 9:100 ("timeout in ms (-1)"), 11:w319) -> (0:w321:errorcluster, 3:w320:refnum<k21>)  [unwired: 1 in, 1 out]
              n97 = Destroy Stream Endpoint(8:w321, 11:w320) -> (0:w314:errorcluster)
            }
          }
        }
        frame Enabled {
        }
      }
      n98 = property on="Sampling\nFrequency" class="DigNum (strict)"(error in=w121) -> ("Value"=w122:dbl)  [unwired: 1 in, 2 out]
      n99 = Get Date/Time In Seconds "Start Time\nIn Seconds"() -> (seconds since 1Jan1904=w126:timestamp)
      "start time" <- w126
      n100 = Tick Count (ms)() -> (millisecond timer value=w131:u32)
      n101 = local read "start time"() -> (w120:timestamp)
      n102 = call "build_labels.vi"("Labels for saving"=w73, "Analog Data Array In"=w72) -> ("Labels"=w88:string[][], "Label Indicies"=w87:i32[])  [unwired: 8 in]
      n103 = property on="Offsets" class="Arr (strict)"(error in=w79) -> ("Value"=w115:T26)  [unwired: 1 in, 2 out]
      n104 = property on="Data Labels" class="Arr (strict)"("Value"=w88) -> ()  [unwired: 2 in, 2 out]
      n105 = call <vilib>:"DAQmx Start Task.vi"("task/channels in"=w114, "error in"=w113) -> ("task out"=w106:refnum<k21>, "error out"=w105:errorcluster)  [unwired: 12 in]
      n106 = while {
        stop <- w485 stop-if-true
        # "Disables Setpoint/Voltage for Manual/PID modes"
        n107 = local read "Stop"() -> (w485:bool)
        n108 = event shown="[0] Timeout" {
          selector: _ -> [_ _ _]
          dyn-events: _ -> [_ _ _]
          timeout: 50 -> [_ _ _]
          event Timeout {
            n109 = event-data() -> ()  [unwired: 1 in, 3 out]
          }
          event Value Change {
            n110 = event-data() -> ("NewVal"=w487:bool)  [unwired: 1 in]
            n111 = case shown="False" w487 {
              frame False {
                n112 = control-ref of="Valve Voltage [V]"() -> (w491:refnum<vi>)
                n113 = property class="DigNum (strict)"(reference=w491, "DisabledEnum"=T28."Enabled" ("Disabled")) -> ()  [unwired: 1 in, 2 out]
                n114 = control-ref of="Flow Set Point [g/s]"() -> (w489:refnum<vi>)
                n115 = property class="DigNum (strict)"(reference=w489, "DisabledEnum"=T28."Disabled and Grayed Out" ("Disabled")) -> ()  [unwired: 1 in, 2 out]
              }
              frame True {
                n116 = property on="Valve Voltage [V]" class="DigNum (strict)"("DisabledEnum"=T28."Disabled and Grayed Out" ("Disabled")) -> ()  [unwired: 2 in, 2 out]
                n117 = property on="Flow Set Point [g/s]" class="DigNum (strict)"("DisabledEnum"=T28."Enabled" ("Disabled")) -> ()  [unwired: 2 in, 2 out]
              }
            }
          }
          event Value Change {
            n118 = event-data() -> ("NewVal"=w494:bool)  [unwired: 1 in]
            n119 = case shown="False" w494 {
              frame False {
                n120 = control-ref of="Valve Voltage [V]"() -> (w498:refnum<vi>)
                n121 = property class="DigNum (strict)"(reference=w498, "DisabledEnum"=T28."Enabled" ("Disabled")) -> ()  [unwired: 1 in, 2 out]
                n122 = control-ref of="Flow Set Point [g/s]"() -> (w496:refnum<vi>)
                n123 = property class="DigNum (strict)"(reference=w496, "DisabledEnum"=T28."Disabled and Grayed Out" ("Disabled")) -> ()  [unwired: 1 in, 2 out]
              }
              frame True {
                n124 = control-ref of="Valve Voltage [V]"() -> (w502:refnum<vi>)
                n125 = control-ref of="Flow Set Point [g/s]"() -> (w501:refnum<vi>)
                n126 = property class="DigNum (strict)"(reference=w501, "DisabledEnum"=T28."Enabled" ("Disabled")) -> ()  [unwired: 1 in, 2 out]
                n127 = property class="DigNum (strict)"(reference=w502, "DisabledEnum"=T28."Disabled and Grayed Out" ("Disabled")) -> ()  [unwired: 1 in, 2 out]
              }
            }
          }
        }
      }
      n128 = disable-structure shown="Enabled" {
        frame Disabled {
        }
        frame Enabled {
          # "Test Section Window Heater Safety Trigger"
          n129 = control-ref of="Flow rate [g/s]"() -> (w433:refnum<vi>)
          n130 = control-ref of="Flow rate [g/s]"() -> (w432:refnum<vi>)
          n131 = control-ref of="Window Heater Switch"() -> (w436:refnum<vi>)
          n132 = control-ref of="Safety Trigger"() -> (w437:refnum<vi>)
          n133 = control-ref of="Stop"() -> (w434:refnum<vi>)
          n134 = control-ref of="Minimum Test Section Mass Flow"() -> (w435:refnum<vi>)
          n135 = call "windows_heater_safety.vi"("Stop!"=w434, "Minimum Flow Rate Refnum"=w435, "Liquid Flow Rate Refnum"=w432, "Vapor Flow Rate Refnum"=w433, "Safety Trigger Refnum"=w437, "Switch Refnum"=w436) -> ()  [unwired: 1 in]
        }
      }
      n136 = disable-structure shown="Enabled" {
        frame Enabled {
          # "Pulse Generator Safety Triggers"
          n137 = local read "Input"() -> (w468:T15)
          n138 = control-ref of="Float 1"() -> (w484:refnum<vi>)
          n139 = control-ref of="Float 2"() -> (w482:refnum<vi>)
          n140 = control-ref of="Float 3"() -> (w481:refnum<vi>)
          n141 = control-ref of="Float 4"() -> (w483:refnum<vi>)
          n142 = control-ref of="Float 5"() -> (w471:refnum<vi>)
          n143 = Unbundle By Name(w468) -> ("Float Switch Line Mode"=w467:bool)
          n144 = Unbundle By Name(w468) -> ("Float Switch Physical Channels"=w470:T13)
          n145 = Build Array(w484, w482, w481, w483, w471) -> (w480:refnum<vi>[])
          n146 = control-ref of="Heaters"() -> (w477:refnum<vi>)
          n147 = control-ref of="Stop"() -> (w478:refnum<vi>)
          n148 = control-ref of="Seconds Allowed Pulse Generator Excess Pressure"() -> (w474:refnum<vi>)
          n149 = control-ref of="TS Temperature W1"() -> (w472:refnum<vi>)
          n150 = control-ref of="PG Abs Pressure"() -> (w476:refnum<vi>)
          n151 = control-ref of="Pulse Generator"() -> (w479:refnum<vi>)
          n152 = control-ref of="Absolute Pulse Generator Pressure Limit"() -> (w475:refnum<vi>)
          n153 = control-ref of="Absolute Pulse Generator Temperature Limit"() -> (w473:refnum<vi>)
          n154 = Cluster To Array(cluster=w470) -> (array=w469:tag[])
          n155 = call "float_switch_check.vi"("Temperature Refnum"=w472, "Heater Refnum"=w477, "Abs Pressure Refnum"=w476, "InvertLines"=w467, "Abs Temperature Limit Refnum"=w473, "Timeout Refnum"=w474, "Abs Pressure Limit Refnum"=w475, "STOP! Refnum"=w478, "Pulse Generator Slide Refnum"=w479, "Float Indicator Refnum"=w480, "lines array"=w469) -> ()
        }
        frame Disabled {
        }
      }
      n156 = disable-structure shown="Enabled" {
        frame Disabled {
        }
        frame Enabled {
          # "Test Section Window Heater Switch"
          n157 = local read "Output"() -> (w431:T19)
          n158 = Unbundle By Name(w431) -> ("Window Heaters Physical Channels.On/Off"=w428:tag)
          n159 = control-ref of="Window Heater Switch"() -> (w430:refnum<vi>)
          n160 = control-ref of="Stop"() -> (w429:refnum<vi>)
          n161 = call "windows_heater.vi"("Stop! Refnum"=w429, "Switch Refnum"=w430, "Window Heater Switch"=w428) -> ()  [unwired: 1 in]
        }
      }
      n162 = while {
        tunnel: w106 -> [w250]
        tunnel: w105 -> [w249]
        shift-right: [w242] -> _
        shift-left: w131 -> [w243]
        tunnel: w126 -> [w245]
        tunnel: [w232] -> w108
        tunnel: [w233] -> w107
        shift-right: [w238] -> _
        shift-left: w122 -> [w239]
        shift-right: [w234] -> _
        shift-left: w124 -> [w235]
        tunnel: w120 -> [w231]
        shift-right: [w228] -> _
        shift-left: w72 -> [w175]
        tunnel: w118 -> [w206]
        shift-right: [w177] -> _
        shift-left: w115 -> [w229]
        tunnel: w87 -> [w184]
        i -> [w247]
        stop <- w248 stop-if-true
        n163 = local read "Stop"() -> (w248:bool)
        n164 = Get Date/Time In Seconds "Iteration\nStart Time"() -> (seconds since 1Jan1904=w246:timestamp)
        "Time Stamp" <- w246
        n165 = call "loop_time.vi"("previous timer value"=w243) -> ("millisecond timer value"=w242:u32, "Loop Time [ms]"=→"Loop Time [ms]":u32)
        n166 = Subtract(x=w246, y=w245) -> (x-y=→"Seconds Since\nSession Start":dbl)
        n167 = call-poly <vilib>:"DAQmx Read.vi"("task/channels in"=w250, "number of samples per channel"=w235, "error in"=w249) -> ("task out"=w236:refnum<k21>, "data"=w174:waveform(dbl)[], "error out"=w230:errorcluster)  [unwired: 10 in]
        n168 = call "data_processor.vi"("Active Analog Data Packages In"=w175, "start time"=w231, "data"=w174, "error in"=w230) -> ("Analog Data Array"=w179:T39[], "timestamp"=w201:dbl[], "error out"=w200:errorcluster)  [unwired: 9 in]
        n169 = property on="Pressure/Temperature/Mixture Properties" class="Clust (strict)"(error in=w230) -> ("Value"=w207:T2)  [unwired: 1 in, 2 out]
        n170 = call "data_distributor_naive.vi"("error in"=w200, "Indicies"=w206, "Analog Data Array In"=w179) -> ("error out"=w197:errorcluster, "Pressure/Temperature/Mixture Properties"=w183:T2, "Measurements Data"=w182:T8, "Liquid Flow"=w195:cluster{"Average":dbl, "Average":dbl}, "Diode Charts"=w198:T10, "Vapor Flow"=w196:cluster{"Average":dbl, "Average":dbl}, "Pulse Generator Charts"=w199:T9)  [unwired: 2 in]
        n171 = local read "autoOffsetPsatQueue"() -> (w211:refnum<queue>)
        n172 = property on="Liquid Flow" class="Clust (strict)"("Value"=w195) -> ()  [unwired: 2 in, 2 out]
        n173 = property on="Vapor Flow" class="Clust (strict)"("Value"=w196) -> ()  [unwired: 2 in, 2 out]
        n174 = local write "Pulse Generator Charts"(w199) -> ()
        n175 = local write "Diode Charts"(w198) -> ()
        n176 = control-ref of="Auto Offset"() -> (w210:refnum<vi>)
        n177 = property on="Sampling\nFrequency" class="DigNum (strict)"() -> ("Value"=w237:dbl)  [unwired: 2 in, 2 out]
        n178 = control-ref of="Auto Offset Progress"() -> (w208:refnum<vi>)
        n179 = call "brians_diode_screen.vi"("Diode Charts In"=w198) -> ()
        n180 = local write "Measurements Data"(w182) -> ()
        n181 = local write "Pressure/Temperature/Mixture Properties"(w183) -> ()
        n182 = property on="Power [W]" class="DigNum (strict)"(error in=w197) -> (error out=w193:errorcluster, "Value"=w180:dbl)  [unwired: 1 in, 1 out]
        n183 = Equal?(x=w239, y=w237) -> (x = y?=w240:bool)
        n184 = call "enqueue_pressure_auto_offset.vi"("autoOffsetPsatQueue"=w211, "# to average"=30.0, "Auto Offset"=w210, "Pressure/Temperature/Mixture Properties"=w207, "Auto Offset ProgressBar"=w208) -> ()
        n185 = case shown="True" w240 {
          tunnel: w239 -> [_ w273]
          tunnel: [w265 w273] -> w238
          tunnel: w237 -> [w265 _]
          tunnel: w236 -> [w269 w272]
          tunnel: w230 -> [w268 w271]
          tunnel: [w261 w272] -> w233
          tunnel: [w260 w271] -> w232
          tunnel: w235 -> [_ w270]
          tunnel: [w259 w270] -> w234
          frame False {
            n186 = call <vilib>:"DAQmx Stop Task.vi"("task/channels in"=w269, "error in"=w268) -> ("task out"=w267:refnum<k21>, "error out"=w266:errorcluster)  [unwired: 12 in]
            n187 = Divide(x=w265, y=10.0) -> (x/y=w259:dbl)
            n188 = property class="DAQmx Timing"(reference=w267, error in=w266, "SampClk.Rate"=w265, "SampQuant.SampPerChan"=w259) -> (reference out=w263:refnum<k21>, error out=w262:errorcluster)
            n189 = call <vilib>:"DAQmx Start Task.vi"("task/channels in"=w263, "error in"=w262) -> ("task out"=w261:refnum<k21>, "error out"=w260:errorcluster)  [unwired: 12 in]
          }
          frame True {
          }
        }
        n190 = property on="Liquid PID Control" class="Clust (strict)"(error in=w230) -> (error out=w212:errorcluster, "Value"=w220:T5)  [unwired: 1 in, 1 out]
        n191 = property on="Vapor PID Control" class="Clust (strict)"(error in=w212) -> ("Value"=w221:T5)  [unwired: 1 in, 2 out]
        n192 = local read "Pulse Train, Steam Heater Controls"() -> (w214:T23)
        n193 = local read "Loop Time [ms]"() -> (w213:u32)
        n194 = Unbundle By Name(w220) -> ("Flow Set Point [g/s]"=w226:dbl, "Flow.Flow rate [g/s]"=w225:dbl)
        n195 = Unbundle By Name(w221) -> ("Flow Set Point [g/s]"=w224:dbl, "Flow.Flow rate [g/s]"=w223:dbl)
        n196 = local read "Data Saving Parameters"() -> (w190:T25)
        n197 = Unbundle By Name(w214) -> ("Valve Voltage [V]"=w205:dbl, "Valve On/Off"=w204:bool)
        n198 = call "valve_control.vi"("Loop Time [ms]"=w213, "PID Control"=w221) -> ("Valve Voltage [V]"=w218:dbl, "PID Control Output"=w216:T5)  [unwired: 1 in]
        n199 = call "valve_control.vi"("Loop Time [ms]"=w213, "PID Control"=w220) -> ("Valve Voltage [V]"=w217:dbl, "PID Control Output"=w215:T5)  [unwired: 1 in]
        n200 = Bundle("Flow Set Point [g/s]"=w224, "Flow rate [g/s]"=w223) -> (→"Vapor Mass Flow Rate":T6)  [unwired: 1 in]
        n201 = Bundle("Flow Set Point [g/s]"=w226, "Flow rate [g/s]"=w225) -> (→"Liquid Mass Flow Rate":T6)  [unwired: 1 in]
        n202 = local write "Vapor PID Control"(w216) -> ()
        n203 = local write "Liquid PID Control"(w215) -> ()
        n204 = Unbundle By Name(w190) -> ("Sampling\nFrequency"=w192:dbl, "Recording Duration [s]"=w191:dbl)
        n205 = Select(t=w205, s=w204, f=1.0) -> (s? t:f=w202:dbl)
        n206 = Build Array(w218, w217, w202) -> (→"Valve Voltage Output":dbl[])
        n207 = local read "dataQueue"() -> (w189:refnum<queue>)
        n208 = call "edit_entry.vi"("error in"=w193, "Average"=w180, "Label"="Power", "Active Analog Data In"=w179) -> ("error out"=w194:errorcluster, "Active Analog Data Out"=w178:T39[])  [unwired: 5 in]
        n209 = control-ref of="Record Data"() -> (w188:refnum<vi>)
        n210 = Multiply(x=w192, y=w191) -> (x*y=w186:dbl)
        n211 = control-ref of="Data Recording Progress"() -> (w187:refnum<vi>)
        n212 = call "enqueue_data.vi"("Active Analog Data In"=w178, "Label indicies In"=w184, "timestamp"=w201, "# of Samples"=w186, "error in"=w194, "data Queue"=w189, "Record dP Data"=w188, "dP Recording Progress"=w187) -> ("error out"=w176:errorcluster)  [unwired: 7 in]
        n213 = property on="Offsets" class="Arr (strict)"(error in=w176) -> ("Value"=w177:T26)  [unwired: 1 in, 2 out]
        n214 = Not Equal?(x=w177, y=w229) -> (x != y?=w185:bool)
        n215 = case shown="True" w185 {
          tunnel: w178 -> [w251 w252]
          tunnel: [w251 w253] -> w228
          frame False {
          }
          frame True {
            n216 = for {
              tunnel: "Offsets" -> [w257] mode=indexing
              tunnel: [w258] -> w253 mode=indexing
              tunnel: w252 -> [w255] mode=indexing
              n217 = Unbundle By Name(w257) -> ("Offset"=w256:dbl)
              n218 = Bundle By Name(cluster=w255, "Offset"=w256) -> (w258:T39)
            }
          }
        }
        "# of Datasets Processed" <- w247
      }
      n219 = while {
        tunnel: w73 -> [w133]
        tunnel: w72 -> [w132]
        stop <- w134 stop-if-true
        n220 = event shown="[1] \"Generate MATLAB Parsing Script\": Value Change" {
          selector: _ -> [_ _]
          dyn-events: _ -> [_ _]
          timeout: _ -> [_ _]
          tunnel: [TRUE _] -> w134
          tunnel: w133 -> [_ w137]
          tunnel: w132 -> [_ w136]
          event Timeout; "Stop": Value Change {
            n221 = event-data() -> ()  [unwired: 1 in, 3 out]
          }
          event "Generate MATLAB Parsing Script": Value Change {
            n222 = event-data() -> ("NewVal"=w138:bool)  [unwired: 1 in]
            n223 = case shown="True" w138 {
              tunnel: w137 -> [_ w142]
              tunnel: w136 -> [_ w141]
              frame False {
              }
              frame True {
                n224 = property on="Data Folder" class="Path"() -> ("Value"=w140:path)  [unwired: 2 in, 2 out]
                n225 = call "File Dialog"("start path"=w140) -> ("selected path"=w139:path)  [unwired: 11 in, 3 out]
                n226 = call "build_labels.vi"("MATLAB File Directory"=w139, "Save MATLAB Parser?"=TRUE, "Labels for saving"=w142, "Analog Data Array In"=w141) -> ()  [unwired: 6 in, 2 out]
              }
            }
          }
        }
      }
      n227 = disable-structure shown="Enabled" {
        frame Disabled {
        }
        frame Enabled {
          w449 = T44 {"Start Pulse"=refnum, "Stop Pulse"=refnum, "Heaters"=refnum, "Counter"=refnum, "Frequency (Hz)"=refnum, "Duty Cycle"=refnum, "Idle State"=refnum, "Pulse Generator Active"=refnum, "Stepper Motor Direction"=refnum, "Steps"=refnum, "Direction Line"=refnum, "1000-1 Line"=refnum, "1000-2 Line"=refnum, "1000-3 Line"=refnum, "500-1 Line"=refnum, "250-1 Line"=refnum, "1000-1"=refnum, "1000-2"=refnum, "1000-3"=refnum, "500-1"=refnum, "250-1"=refnum, "150-1"=refnum, "Heater ON?"=refnum, "150-1 Line"=refnum, "Power"=refnum}  # Pulse Generator Control Refnums
          # "Controls Heaters and Stepper Motor, listens to stopping signals."
          n228 = control-ref of="Counter Line"() -> (w440:refnum<vi>)
          n229 = control-ref of="Direction Line"() -> (w441:refnum<vi>)
          n230 = control-ref of="1000W 1"() -> (w459:refnum<vi>)
          n231 = control-ref of="1000W 2"() -> (w465:refnum<vi>)
          n232 = control-ref of="1000W 3"() -> (w460:refnum<vi>)
          n233 = control-ref of="500W 1"() -> (w461:refnum<vi>)
          n234 = control-ref of="250W 1"() -> (w462:refnum<vi>)
          n235 = control-ref of="150W 1"() -> (w448:refnum<vi>)
          n236 = control-ref of="Start Pulse"() -> (w455:refnum<vi>)
          n237 = control-ref of="Stop Pulse"() -> (w454:refnum<vi>)
          n238 = control-ref of="Heaters"() -> (w450:refnum<vi>)
          n239 = control-ref of="Pulse Gen\nActive?"() -> (w452:refnum<vi>)
          n240 = control-ref of="Stepper Motor Direction"() -> (w451:refnum<vi>)
          n241 = control-ref of="Heater ON?"() -> (w458:refnum<vi>)
          n242 = control-ref of="1000-1"() -> (w464:refnum<vi>)
          n243 = control-ref of="1000-2"() -> (w463:refnum<vi>)
          n244 = control-ref of="1000-3"() -> (w466:refnum<vi>)
          n245 = control-ref of="500-1"() -> (w447:refnum<vi>)
          n246 = control-ref of="250-1"() -> (w446:refnum<vi>)
          n247 = control-ref of="150-1"() -> (w445:refnum<vi>)
          n248 = control-ref of="Power [W]"() -> (w439:refnum<vi>)
          n249 = control-ref of="Frequency (Hz)"() -> (w453:refnum<vi>)
          n250 = control-ref of="Duty Cycle"() -> (w444:refnum<vi>)
          n251 = control-ref of="Steps"() -> (w443:refnum<vi>)
          n252 = control-ref of="Idle State"() -> (w442:refnum<vi>)
          n253 = Bundle By Name(cluster=w449, "Start Pulse"=w455, "Stop Pulse"=w454, "Heaters"=w450, "Counter"=w440, "Frequency (Hz)"=w453, "Duty Cycle"=w444, "Steps"=w443, "Idle State"=w442, "Pulse Generator Active"=w452, "Stepper Motor Direction"=w451, "Direction Line"=w441, "Heater ON?"=w458, "1000-1 Line"=w459, "1000-2 Line"=w465, "1000-3 Line"=w460, "500-1 Line"=w461, "250-1 Line"=w462, "150-1 Line"=w448, "1000-1"=w464, "1000-2"=w463, "1000-3"=w466, "500-1"=w447, "250-1"=w446, "150-1"=w445, "Power"=w439) -> (w456:T44)
          n254 = control-ref of="Stop"() -> (w457:refnum<vi>)
          n255 = call "pulse_generator_multiheater_refnum.vi"("Stop! Refnum"=w457, "Pulse Generator Control Multiheater Refnums"=w456) -> ()  [unwired: 2 in]
        }
      }
      n256 = while {
        stop <- w503 stop-if-true
        # "Dequeue loop for auto offset function"
        n257 = event shown="[1] \"Auto Offset\": Value Change" {
          selector: _ -> [_ _]
          dyn-events: _ -> [_ _]
          timeout: _ -> [_ _]
          tunnel: [TRUE _] -> w503
          event Timeout; "Stop": Value Change {
            n258 = event-data() -> ()  [unwired: 1 in, 3 out]
          }
          event "Auto Offset": Value Change {
            n259 = event-data() -> ("NewVal"=w506:bool)  [unwired: 1 in]
            n260 = case shown="False" w506 {
              frame False {
                n261 = local read "autoOffsetPsatQueue"() -> (w535:refnum<queue>)
                n262 = Initialize Array(0.0 ("element"), 8 ("dimension size")) -> (w514:dbl[])
                n263 = while {
                  tunnel: w535 -> [w543]
                  shift-right: [w538] -> w534
                  shift-left: w514 -> [w539]
                  tunnel: [w537] -> w532
                  i -> [w537]
                  stop <- w541 stop-if-true
                  n264 = Dequeue Element(queue=w543, timeout in ms (-1)=500) -> (element=w540:dbl[], timed out?=w542:bool)  [unwired: 1 in, 2 out]
                  n265 = case shown="False" w542 {
                    selector: w542 -> [_ w551]
                    tunnel: [w544 w551] -> w541
                    tunnel: w540 -> [w548 _]
                    tunnel: [w547 w550] -> w538
                    tunnel: w539 -> [w549 w550]
                    frame False {
                      n266 = local read "Stop"() -> (w545:bool)
                      n267 = Add(x=w549, y=w548) -> (x+y=w547:dbl[])
                      n268 = Or(x=w545, y=FALSE) -> (x .or. y?=w544:bool)
                    }
                    frame True {
                    }
                  }
                }
                n269 = property on="Offset Parameters" class="Clust (strict)"() -> ("Value"=w508:T3)  [unwired: 2 in, 2 out]
                n270 = Add(x=w532, y=1) -> (x+y=w533:i32)
                n271 = Divide(x=w534, y=w533) -> (x/y=w530:dbl[])
                n272 = Unbundle By Name(w508) -> ("Liquid Tank\nPressure"=w528:dbl, "Separator Pressure"=w527:dbl, "Liquid Inlet\nPressure"=w521:dbl, "Vapor Tank\nPressure"=w526:dbl, "Vapor Inlet\nPressure"=w522:dbl, "Test Section\nPressure"=w525:dbl, "Upper Dev Section\nPressure"=w524:dbl, "Lower Dev Section\nPressure"=w509:dbl)
                n273 = Build Array(w528, w527, w521, w526, w522, w525, w524, w509) -> (w523:dbl[])
                n274 = Subtract(x=w530, y=w523) -> (x-y=w529:dbl[])
                n275 = Index Array(array=w529) -> (element #1=w520:dbl, element #2=w519:dbl, element #3=w518:dbl, element #4=w517:dbl, element #5=w513:dbl, element #6=w512:dbl, element #7=w511:dbl, element #8=w510:dbl)  [unwired: 8 in]
                n276 = Bundle By Name(cluster=w508, "Liquid Tank\nPressure"=w520, "Separator Pressure"=w519, "Liquid Inlet\nPressure"=w518, "Vapor Tank\nPressure"=w517, "Vapor Inlet\nPressure"=w513, "Test Section\nPressure"=w512, "Upper Dev Section\nPressure"=w511, "Lower Dev Section\nPressure"=w510) -> (w507:T3)
                n277 = property on="Offset Parameters" class="Clust (strict)"("Val(Sgnl)"=w507) -> ()  [unwired: 2 in, 2 out]
              }
              frame True {
                n278 = property on="Offset Parameters" class="Clust (strict)"("DisabledEnum"=T28."Disabled and Grayed Out" ("Disabled")) -> ()  [unwired: 2 in, 2 out]
              }
            }
            n279 = property on="Offset Parameters" class="Clust (strict)"("DisabledEnum"=T28."Enabled" ("Disabled")) -> ()  [unwired: 2 in, 2 out]
          }
        }
      }
      n280 = while {
        tunnel: [w286] -> w112
        tunnel: [w285] -> w89
        stop <- w287 continue-if-true
        n281 = property on="# of Datasets Processed" class="DigNum (strict)"() -> (error out=w286:errorcluster, "Value"=w289:i32)  [unwired: 2 in, 1 out]
        n282 = Less?(x=w289, y=1) -> (x < y?=w287:bool)
        n283 = local read "Offsets"() -> (w285:T26)
      }
      n284 = Array Size(array=w110) -> (size(s)=w111:i32)
      n285 = for {
        N: w111 -> [_]
        tunnel: w110 -> [w278] mode=indexing
        tunnel: w112 -> [_]
        tunnel: w89 -> [w279]
        tunnel: [w274] -> w109 mode=indexing
        n286 = for {
          tunnel: w279 -> [w284] mode=indexing
          tunnel: w278 -> [w282]
          tunnel: [w281] -> w276
          tunnel: [w280] -> w277
          i -> [w281]
          stop <- w280 stop-if-true
          n287 = Unbundle(w284) -> ("Channel"=w283:string)  [unwired: 2 out]
          n288 = Equal?(x=w283, y=w282) -> (x = y?=w280:bool)
        }
        n289 = Select(t=w276, s=w277, f=-1) -> (s? t:f=w274:i32)
      }
      n290 = while {
        stop <- w403 stop-if-true
        # "Updates Visual Loop Data Display (low priority)"
        n291 = local read "Pressure/Temperature/Mixture Properties"() -> (w427:T2)
        n292 = local read "Measurements Data"() -> (w411:T8)
        n293 = Unbundle By Name(w427) -> ("Component PTs"=w426:T45, "Ambient Pressure [Pa]"=w412:dbl)
        n294 = local read "Liquid PID Control"() -> (w399:T5)
        n295 = local read "Vapor PID Control"() -> (w398:T5)
        n296 = Wait (ms)(milliseconds to wait=u32 500) -> ()  [unwired: 1 out]
        n297 = Unbundle By Name(w411) -> ("PG Abs Pressure"=w410:dbl, "PG Mass Flow Rate"=w409:dbl, "Vapor Temperature"=w408:dbl, "Liquid Temperature"=w407:dbl, "W1-4 dP[Pa]"=w406:dbl, "W1-7 dP[Pa]"=w405:dbl)
        n298 = Unbundle By Name(w426) -> ("Liquid Tank P"=w424:dbl, "Liquid Tank T"=w423:dbl, "Separator P"=w422:dbl, "Separator T"=w421:dbl, "Liquid Inlet P"=w420:dbl, "Liquid Inlet T"=w419:dbl, "Vapor Tank P"=w418:dbl, "Vapor Tank T"=w417:dbl, "Vapor Inlet P"=w416:dbl, "Vapor Inlet T"=w415:dbl, "Upper Dev Section P"=w414:dbl, "Lower Dev Section P"=w413:dbl)
        n299 = Unbundle By Name(w398) -> ("Flow.Flow rate [g/s]"=w402:dbl)
        n300 = Unbundle By Name(w399) -> ("Flow.Flow rate [g/s]"=w401:dbl)
        n301 = local read "Visual Loop Display"() -> (w425:T4)
        n302 = Bundle By Name(cluster=w425, "LiqTkPres"=w424, "LiqTkTemp"=w423, "SepPres"=w422, "SepTemp"=w421, "LiqInPres"=w420, "LiqInTemp"=w419, "VpTkPres"=w418, "VpTkTemp"=w417, "VapInPres"=w416, "VapInTemp"=w415, "TSInPres"=w414, "TSInTemp"=w413, "TSPres"=w412, "PgPres"=w410, "PGMass"=w409, "PGVapTemp"=w408, "PGLiqTemp"=w407, "Win1-4dP"=w406, "Win1-7dP"=w405, "VpMass"=w402, "LiqMass"=w401) -> (→"Visual Loop Display":T4)
        n303 = local read "Stop"() -> (w403:bool)
      }
      n304 = while {
        shift-right: [w291] -> _
        shift-left: w109 -> [w290]
        stop <- w294 stop-if-true
        n305 = event shown="[1] \"Offset Parameters\": Value Change" {
          selector: _ -> [_ _]
          dyn-events: _ -> [_ _]
          timeout: _ -> [_ _]
          tunnel: [TRUE _] -> w292
          tunnel: w290 -> [w295 w297]
          tunnel: [w295 w297] -> w291
          event Timeout; "Stop": Value Change {
            n306 = event-data() -> ()  [unwired: 1 in, 3 out]
          }
          event Value Change {
            n307 = event-data() -> ("NewVal"=w299:T3)  [unwired: 1 in]
            n308 = Cluster To Array(cluster=w299) -> (array=w298:dbl[])
            n309 = for {
              tunnel: w298 -> [w302] mode=indexing
              tunnel: w297 -> [w305] mode=indexing
              n310 = local read "Offsets"() -> (w303:T26)
              n311 = Index Array(array=w303, index=w305) -> (element=w304:T46)
              n312 = Bundle By Name(cluster=w304, "Offset"=w302) -> (w301:T46)
              n313 = Replace Array Subset(array=w303, new element=w301, index=w305) -> (w300:T26)
              n314 = local write "Offsets"(w300) -> ()
            }
          }
        }
        n315 = local read "Stop"() -> (w293:bool)
        n316 = Or(x=w292, y=w293) -> (x .or. y?=w294:bool)
      }
      n317 = local read "dataQueue"() -> (w127:refnum<queue>)
      n318 = while {
        tunnel: w127 -> [w622]
        tunnel: [w618] -> _
        stop <- w619 stop-if-true
        # "Dequeue loop of data logging"
        n319 = Dequeue Element(queue=w622, timeout in ms (-1)=50) -> (queue out=w618:refnum<queue>, element=w620:dbl[][], timed out?=w617:bool)  [unwired: 1 in, 1 out]
        n320 = case shown="False" w617 {
          tunnel: w620 -> [w627 _]
          frame False {
            n321 = property on="Data Prefix" class="Str"() -> ("Value"=w625:string)  [unwired: 2 in, 2 out]
            n322 = property on="Data Folder" class="Path"() -> ("Value"=w626:path)  [unwired: 2 in, 2 out]
            n323 = local read "Data Labels"() -> (w623:string[][])
            n324 = property on="Data Index" class="DigNum (strict)"() -> ("Value"=w624:i32)  [unwired: 2 in, 2 out]
            n325 = call "write_data.vi"("Data Folder"=w626, "dP Data Prefix"=w625, "dP Data Index"=w624, "Data Labels"=w623, "dequeued data"=w627) -> ()  [unwired: 1 in]
          }
          frame True {
          }
        }
        n326 = local read "Stop"() -> (w619:bool)
      }
      n327 = while {
        tunnel: w127 -> [w554]
        stop <- w553 stop-if-true
        # "Makes sure the path and daq settings cannot be changed while data is being recorded."
        n328 = event shown="[1] \"Data Saving Parameters.Record Data\": Value Change" {
          selector: _ -> [_ _]
          dyn-events: _ -> [_ _]
          timeout: _ -> [_ _]
          tunnel: w554 -> [_ w557]
          tunnel: [TRUE _] -> w553
          event Timeout; "Stop": Value Change {
            n329 = event-data() -> ()  [unwired: 1 in, 3 out]
          }
          event "Data Saving Parameters.Record Data": Value Change {
            n330 = event-data() -> ("NewVal"=w556:bool)  [unwired: 1 in]
            n331 = case shown="False" w556 {
              tunnel: w557 -> [w559 _]
              frame False {
                n332 = flat-sequence {
                  tunnel: w559 -> [w561]
                  tunnel: [w570] -> w558
                  tunnel: w558 -> [w594]
                  frame #0 {
                    n333 = while {
                      tunnel: w561 -> [w562]
                      stop <- w563 stop-if-true
                      n334 = Get Queue Status(queue=w562) -> (# elements in queue=w567:i32)  [unwired: 2 in, 7 out]
                      n335 = local read "Stop"() -> (w564:bool)
                      n336 = Equal?(x=0, y=w567) -> (x = y?=w565:bool)
                      n337 = Or(x=w565, y=w564) -> (x .or. y?=w563:bool)
                    }
                    n338 = property on="Record Data" class="Bool (strict)"("DisabledEnum"=T28."Disabled and Grayed Out" ("Disabled")) -> ()  [unwired: 2 in, 2 out]
                  }
                  frame #1 {
                    n339 = Wait (ms)(milliseconds to wait=u32 1000) -> ()  [unwired: 1 out]
                  }
                  frame #2 {
                    w581 = T47 5 items=["User Home"=0, "User Desktop"=1, "User Documents"=2, "User Application Data"=3, "User Preferences"=4, "User Temporary"=5, "Public Documents"=6, "Public Application Data"=7, "Public Preferences"=8, "Public Cache"=13, "System Core Libraries"=9, "System Installed Libraries"=10, "Application Files"=11, "Boot Volume Root"=12] ("system directory type")
                    n340 = property on="Notes:" class="Str"() -> ("Value"=w571:string)  [unwired: 2 in, 2 out]
                    n341 = property on="Data Index" class="DigNum (strict)"() -> ("Value"=w589:i32)  [unwired: 2 in, 2 out]
                    n342 = property on="Data Prefix" class="Str"() -> ("Value"=w587:string)  [unwired: 2 in, 2 out]
                    n343 = property on="Data Index" class="DigNum (strict)"() -> ("Value"=w572:i32)  [unwired: 2 in, 2 out]
                    n344 = Format Into String(format string="%04d", w572) -> (resulting string=w574:string)  [unwired: 2 in, 1 out]
                    n345 = call <vilib>:"Get System Directory.vi"("system directory type"=w581) -> ("system directory"=w590:path)  [unwired: 10 in]
                    n346 = Format Into String(format string="%04d%s", initial string="mfval_temp_", w589, ".csv") -> (resulting string=w591:string)  [unwired: 1 in, 1 out]
                    n347 = Format Into String(format string="%04d%s", initial string=w587, w572, ".csv") -> (resulting string=w586:string)  [unwired: 1 in, 1 out]
                    n348 = Bundle(cluster=T34 {"Entry Content"="", "File Number"=""} ("new element/subarray"), "Entry Content"=w574, "File Number"=w571) -> (w575:T34)
                    n349 = property on="Data Folder" class="Path"() -> ("Value"=w585:path)  [unwired: 2 in, 2 out]
                    n350 = Insert Into Array(array="Run Log", new element=w575) -> (w570:T22)  [unwired: 1 in]
                    n351 = Build Path(base path=w590, name or relative path=w591) -> (appended path=w588:path)
                    n352 = Build Path(base path=w585, name or relative path=w586) -> (appended path=w584:path)
                    n353 = Move(source path=w588, 9:TRUE ("overwrite (F)"), 10:w584) -> ()  [unwired: 2 in, 3 out]
                  }
                  frame #3 {
                    w599 = T28."Enabled" ("Disabled")
                    w600 = T28."Enabled" ("Disabled")
                    n354 = local write "Run Log"(w594) -> ()
                    n355 = property on="Data Index" class="DigNum (strict)"() -> (error out=w601:errorcluster, "Value"=w603:i32)  [unwired: 2 in, 1 out]
                    n356 = for {
                      tunnel: w594 -> [w605] mode=indexing
                      tunnel: [w604] -> w593 mode=indexing
                      n357 = Cluster To Array(cluster=w605) -> (array=w604:string[])
                    }
                    n358 = Increment(x=w603) -> (x+1=w602:i32)
                    n359 = property on="Data Index" class="DigNum (strict)"(error in=w601, "Value"=w602) -> ()  [unwired: 1 in, 2 out]
                    n360 = property on="Data Folder" class="Path"("DisabledEnum"=w600) -> ()  [unwired: 2 in, 2 out]
                    n361 = property on="Data Prefix" class="Str"("DisabledEnum"=w600) -> ()  [unwired: 2 in, 2 out]
                    n362 = property on="Data Folder" class="Path"() -> ("Value"=w597:path)  [unwired: 2 in, 2 out]
                    n363 = Format Date/Time String(time format string (%c)="%Y%m%d_log.txt") -> (date/time string=w596:string)  [unwired: 2 in]
                    n364 = Build Path(base path=w597, name or relative path=w596) -> (appended path=w592:path)
                    n365 = call-poly <vilib>:"Write Delimited Spreadsheet.vi"("file path (dialog if empty)"=w592, "2D data"=w593) -> ()  [unwired: 12 in, 2 out]
                    n366 = property on="Record Data" class="Bool (strict)"("DisabledEnum"=w599) -> ()  [unwired: 2 in, 2 out]
                    n367 = property on="Recording Duration [s]" class="DigNum (strict)"("DisabledEnum"=w599) -> ()  [unwired: 2 in, 2 out]
                    n368 = property on="Data Recording Progress" class="Slide (strict)"("Value"=u32 0 ("dP Recording Progress")) -> ()  [unwired: 2 in, 2 out]
                  }
                }
              }
              frame True {
                n369 = control-ref of="Data Folder"() -> (w616:refnum<vi>)
                n370 = control-ref of="Record Data"() -> (w611:refnum<vi>)
                n371 = property class="Path"(reference=w616, "DisabledEnum"=T28."Disabled and Grayed Out" ("Disabled")) -> ()  [unwired: 1 in, 2 out]
                n372 = property class="Bool (strict)"(reference=w611, "DisabledEnum"=T28."Enabled" ("Disabled")) -> ()  [unwired: 1 in, 2 out]
                n373 = control-ref of="Data Prefix"() -> (w613:refnum<vi>)
                n374 = property on="Recording Duration [s]" class="DigNum (strict)"("DisabledEnum"=T28."Disabled and Grayed Out" ("Disabled")) -> ()  [unwired: 2 in, 2 out]
                n375 = property class="Str"(reference=w613, "DisabledEnum"=T28."Disabled and Grayed Out" ("Disabled")) -> ()  [unwired: 1 in, 2 out]
                n376 = property on="Sampling\nFrequency" class="DigNum (strict)"() -> ("Value"=w607:dbl)  [unwired: 2 in, 2 out]
                n377 = property on="Recording Duration [s]" class="DigNum (strict)"() -> ("Value"=w608:dbl)  [unwired: 2 in, 2 out]
                n378 = control-ref of="Data Recording Progress"() -> (w610:refnum<vi>)
                n379 = Multiply(x=w608, y=w607) -> (x*y=w609:dbl)
                n380 = property class="Slide (strict)"(reference=w610, "Scale.Maximum"=w609) -> ()  [unwired: 1 in, 2 out]
              }
            }
          }
        }
      }
      n381 = while {
        stop <- w354 stop-if-true
        # "Partially Reset Offset Values"
        n382 = event shown="[1] \"Zero Pressure Offsets\": Value Change" {
          selector: _ -> [_ _ _]
          dyn-events: _ -> [_ _ _]
          timeout: _ -> [_ _ _]
          tunnel: [TRUE FALSE FALSE] -> w354
          tunnel: [w355 w359 w377] -> w353
          event Timeout; "Stop": Value Change {
            n383 = event-data() -> ()  [unwired: 1 in, 3 out]
            n384 = local read "Offset Parameters"() -> (w355:T3)
          }
          event "Zero Pressure Offsets": Value Change {
            n385 = event-data() -> ("NewVal"=w358:bool)  [unwired: 1 in, 2 out]
            n386 = local read "Offset Parameters"() -> (w357:T3)
            n387 = case shown="True" w358 {
              tunnel: [w361 w366] -> w359
              tunnel: w357 -> [w361 w362]
              frame False {
              }
              frame True {
                n388 = Initialize Array(0.0 ("element"), 8 ("dimension size")) -> (w365:dbl[])
                n389 = Index Array(array=w365) -> (element #1=w367:dbl, element #2=w368:dbl, element #3=w369:dbl, element #4=w370:dbl, element #5=w371:dbl, element #6=w372:dbl, element #7=w373:dbl, element #8=w374:dbl)  [unwired: 8 in]
                n390 = Bundle By Name(cluster=w362, "Liquid Tank\nPressure"=w367, "Separator Pressure"=w368, "Liquid Inlet\nPressure"=w369, "Vapor Tank\nPressure"=w370, "Vapor Inlet\nPressure"=w371, "Test Section\nPressure"=w372, "Upper Dev Section\nPressure"=w373, "Lower Dev Section\nPressure"=w374) -> (w366:T3)
              }
            }
          }
          event "Zero Temp Offsets": Value Change {
            n391 = event-data() -> ("NewVal"=w376:bool)  [unwired: 1 in, 2 out]
            n392 = local read "Offset Parameters"() -> (w375:T3)
            n393 = case shown="True" w376 {
              tunnel: [w379 w384] -> w377
              tunnel: w375 -> [w379 w380]
              frame False {
              }
              frame True {
                n394 = Initialize Array(0.0 ("element"), 7 ("dimension size")) -> (w383:dbl[])
                n395 = Index Array(array=w383) -> (element #1=w385:dbl, element #2=w386:dbl, element #3=w387:dbl, element #4=w388:dbl, element #5=w389:dbl, element #6=w390:dbl, element #7=w391:dbl)  [unwired: 7 in]
                n396 = Bundle By Name(cluster=w380, "Liquid Tank\nTemperature"=w385, "Separator \nTemperature"=w386, "Liquid Inlet\nTemperature"=w387, "Vapor Tank\nTemperature"=w388, "Vapor Inlet \nTemperature"=w389, "Test Section\nTemperature"=w390, "Upper Dev Section\nTemperature"=w391) -> (w384:T3)
              }
            }
          }
        }
        n397 = property on="Offset Parameters" class="Clust (strict)"("Val(Sgnl)"=w353) -> ()  [unwired: 2 in, 2 out]
      }
      n398 = call <vilib>:"DAQmx Stop Task.vi"("task/channels in"=w107, "error in"=w108) -> ("task out"=w128:refnum<k21>, "error out"=w129:errorcluster)  [unwired: 12 in]
      n399 = disable-structure shown="Enabled" {
        frame Enabled {
          # "Valve Output Task"
          n400 = local read "Output"() -> (w397:T19)
          n401 = Unbundle By Name(w397) -> ("Proportional Valve Physical Channels.Vapor Valve"=w396:tag, "Proportional Valve Physical Channels.Liquid Valve"=w395:tag, "Proportional Valve Physical Channels.PG Valve"=w392:tag)
          n402 = control-ref of="Stop"() -> (w394:refnum<vi>)
          n403 = control-ref of="Valve Voltage Output"() -> (w393:refnum<vi>)
          n404 = call "valve_control_output.vi"("STOP! Refnum"=w394, "Voltage Arr Refnum"=w393, "PG channel"=w392, "Liquid channel"=w395, "Vapor channel"=w396) -> ()  [unwired: 1 in]
        }
        frame Disabled {
        }
      }
      n405 = call <vilib>:"DAQmx Clear Task.vi"("task in"=w128, "error in"=w129) -> ("error out"=w130:errorcluster)  [unwired: 13 in]
      n406 = call <vilib>:"Application Directory.vi"() -> ("Application Directory"=w76:path)
      n407 = Build Path(base path=w76, name or relative path="Utility Sub VIs\\brians_diode_screen.vi") -> (appended path=w74:path)
      n408 = Open VI Reference(vi path=w74) -> (vi reference=w93:refnum<vi>, error out=w92:errorcluster)  [unwired: 5 in]
      n409 = while {
        tunnel: w93 -> [w147]
        tunnel: w92 -> [w146]
        tunnel: [w145] -> w91
        tunnel: [w144] -> w90
        stop <- w148 stop-if-true
        n410 = event shown="[0] Timeout;  \"Stop\": Value Change" {
          selector: _ -> [_ _]
          dyn-events: _ -> [_ _]
          timeout: _ -> [_ _]
          tunnel: [TRUE FALSE] -> w148
          tunnel: w147 -> [w155 w168]
          tunnel: w146 -> [w149 w167]
          tunnel: [w157 w166] -> w145
          tunnel: [w156 w165] -> w144
          event Timeout; "Stop": Value Change {
            n411 = event-data() -> ()  [unwired: 1 in, 1 out]
            n412 = property class="VI"(reference=w155, error in=w149) -> (reference out=w151:refnum<vi>, error out=w150:errorcluster, "FP.State"=w153:T33)
            n413 = Equal?(x=w153, y=T33."Closed") -> (x = y?=w154:bool)
            n414 = case shown="True" w154 {
              tunnel: [w160 w164] -> w157
              tunnel: [w159 w163] -> w156
              tunnel: w151 -> [w160 w162]
              tunnel: w150 -> [w159 w161]
              frame True {
              }
              frame False {
                n415 = invoke class="VI" method="FP.Close"(reference=w162, error in=w161) -> (reference out=w164:refnum<vi>, error out=w163:errorcluster)  [unwired: 1 in, 1 out]
              }
            }
          }
          event "Open Brians VI": Value Change {
            n416 = event-data() -> ()  [unwired: 1 in, 1 out]
            n417 = invoke class="VI" method="FP.Open"(reference=w168, error in=w167, "State"=T33."Maximized") -> (reference out=w172:refnum<vi>, error out=w171:errorcluster)  [unwired: 2 in, 3 out]
            n418 = property class="VI" props=["FP.Monitor", "FP.Monitor"](reference=w172, error in=w171, "FP.Monitor"=u16 3 ("Front Panel Window:Monitor")) -> (reference out=w166:refnum<vi>, error out=w165:errorcluster)  [unwired: 1 out]
          }
        }
      }
      n419 = Close Reference(reference=w91, error in (no error)=w90) -> ()  [unwired: 1 out]
    }
    frame #3 {
      w629 = T28."Enabled" ("Disabled")
      n420 = control-ref of="Stop"() -> (w633:refnum<vi>)
      n421 = control-ref of="System Running"() -> (w630:refnum<vi>)
      n422 = property class="Bool (strict)"(reference=w633, "Value"=FALSE) -> ()  [unwired: 1 in, 2 out]
      n423 = property class="Bool (strict)"(reference=w630, "Value"=FALSE) -> ()  [unwired: 1 in, 2 out]
      n424 = property on="Input" class="Clust (strict)"("DisabledEnum"=w629) -> ()  [unwired: 2 in, 2 out]
      n425 = property on="Safety" class="Clust (strict)"("DisabledEnum"=w629) -> ()  [unwired: 2 in, 2 out]
      n426 = property on="Commit Settings" class="Bool (strict)"("DisabledEnum"=w629) -> ()  [unwired: 2 in, 2 out]
      n427 = property on="Output" class="Clust (strict)"("DisabledEnum"=w629) -> ()  [unwired: 2 in, 2 out]
      "error out" <- w628
    }
  }
